vi "record_temp.vi"() -> ()   [LabVIEW 2013]
doc: "Use this template to build a producer/consumer design pattern with events to produce queue items. Use this design pattern instead of the User Interface Event Handler pattern for user interfaces when you want to execute code asynchronously in response to an event without slowing the user interface responsiveness."
uses:
  prog_files_all/ni/labview/examples/Instrument IO/Serial/support/Serial - Settings.ctl
  states_cntrl.ctl
  raw_dat_str.ctl
  temp_ind.ctl
  dts_cntrl.ctl
  rh_ind.ctl
  usr_evnt_main_clstr.ctl
  event_clstr.ctl
  log_dat.ctl
  rh_ind_arry.ctl
  sens_type.ctl
  sens_type_arry_cntrl.ctl
  pibs_clstr.ctl
  sens_type_arry_str_cntrl.ctl
  reg_evnt_ref_clstr.ctl
  labview/power_vi_stm_v13_1_7_22/labview/gen_libs/non_instr/gen_ctls/enums/minor_qsm.ctl
  labview/power_vi_stm_v13_1_7_22/labview/gen_libs/both/gen_ctls/rs232_data_clstr.ctl
  labview/power_vi_stm_v13_1_7_22/labview/gen_libs/non_instr/gen_ctls/enums/state_enum.ctl
  <vilib>/Instr/_visa.llb/VISA Configure Serial Port (Instr).vi
panel:
  out "sens_typ_str _2":T1
  in  "sens_type_8":T2 items=["SHTC3", "SHT3X", "D6T_1A", "HTS221", "AHT20", "ADT7410"]
  in  "sens_type_7":T2 items=["SHTC3", "SHT3X", "D6T_1A", "HTS221", "AHT20", "ADT7410"]
  in  "sens_type_6":T2 items=["SHTC3", "SHT3X", "D6T_1A", "HTS221", "AHT20", "ADT7410"]
  in  "sens_type_5":T2 items=["SHTC3", "SHT3X", "D6T_1A", "HTS221", "AHT20", "ADT7410"]
  in  "sens_type_4":T2 caption="Sensor Type" items=["SHTC3", "SHT3X", "D6T_1A", "HTS221", "AHT20", "ADT7410"]
  in  "sens_type_3":T2 caption="Sensor Type" items=["SHTC3", "SHT3X", "D6T_1A", "HTS221", "AHT20", "ADT7410"]
  in  "sens_type_2":T2 caption="Sensor Type" items=["SHTC3", "SHT3X", "D6T_1A", "HTS221", "AHT20", "ADT7410"]
  in  "sens_type_1":T2 caption="Sensor Type" items=["SHTC3", "SHT3X", "D6T_1A", "HTS221", "AHT20", "ADT7410"]
  out "rh_8":T3 caption="Relative Humidity (%)" format="%#_4g"
  out "sen_8_num":T4 caption="Temp (F)" format="%_4g"
  out "rh_7":T3 caption="Relative Humidity (%)" format="%#_4g"
  out "sen_7_num":T4 caption="Temp (F)" format="%_4g"
  out "rh_6":T3 caption="Relative Humidity (%)" format="%#_4g"
  out "sen_6_num":T4 caption="Temp (F)" format="%_4g"
  out "rh_5":T3 caption="Relative Humidity (%)" format="%#_4g"
  out "sen_5_num":T4 caption="Temp (F)" format="%_4g"
  out "rh_4":T3 caption="Relative Humidity (%)" format="%#_4g"
  out "sen_4_num":T4 caption="Temp (F)" format="%_4g"
  out "sen_3_num":T4 caption="Temp (F)" format="%_4g"
  out "sen_2_num":T4 caption="Temp (F)" format="%_4g"
  out "rh_3":T3 caption="Relative Humidity (%)" format="%#_4g"
  out "rh_2":T3 caption="Relative Humidity (%)" format="%#_4g"
  out "sen_1":T5
  out "sen_1_num":T4 caption="Temp (F)" format="%_4g"
  out "sen_2":T5
  out "sen_3":T5
  out "sen_4":T5
  out "sen_5":T5
  out "sen_6":T5
  out "sen_7":T5
  out "sen_8":T5
  out "rh_1":T3 caption="Relative Humidity (%)" format="%#_4g"
  out "sens_typ_str":T1
  out "sens_type_arry":T6 items=["SHTC3", "SHT3X", "D6T_1A", "HTS221", "AHT20", "ADT7410"]
  in  "regEvntClstr":T7
  in  "user event out":T8
  out "states_ind":T9 caption="State_Ind"
  in  "stop":bool
  in  "tab_cntrl":T10(tab)
  in  "Serial Settings":T11={"baud rate"=19200, "data bits"=8, "parity"=enum."None", "stop bits"=10, "flow control"=0} {"flow control" items=["None"=0, "XON/XOFF"=1, "RTS/CTS"=2, "DTR/DSR"=4]; "stop bits" items=["1.0"=10, "1.5"=15, "2.0"=20]; "data bits" min=5 max=8 step=1; "baud rate" items=["75"=75, "110"=110, "134"=134, "150"=150, "300"=300, "600"=600, "1200"=1200, "1800"=1800, "2400"=2400, "4800"=4800, "7200"=7200, "9600"=9600, "14400"=14400, "19200"=19200, "28800"=28800, "38400"=38400, "56000"=56000, "57600"=57600, "115200"=115200, "128000"=128000, "230400"=230400]}
  in  "VISA resource name":refnum<visa-resource-name>="COM3"
  in  "minor_qsm_qry":bool caption="Use Minor QSM"
  in  "capt_data":bool
  in  "wr_buffr":string="\b"
  in  "dwell_s":u32=60
  in  "auto_capt_data":bool
  in  "delay":u32=10
  out "bytes_at_port":u32
  out "bytes read":u32
  out "Response":string
  in  "small_dwell":u32=3
  in  "chk_bytes_rd":u32=56
  in  "pibs_clstr":T12 {"sens_type_8" items=["SHTC3", "SHT3X", "D6T_1A", "HTS221", "AHT20", "ADT7410"]; "sens_type_7" items=["SHTC3", "SHT3X", "D6T_1A", "HTS221", "AHT20", "ADT7410"]; "sens_type_6" items=["SHTC3", "SHT3X", "D6T_1A", "HTS221", "AHT20", "ADT7410"]; "sens_type_5" items=["SHTC3", "SHT3X", "D6T_1A", "HTS221", "AHT20", "ADT7410"]; "sens_type_4" items=["SHTC3", "SHT3X", "D6T_1A", "HTS221", "AHT20", "ADT7410"]; "sens_type_3" items=["SHTC3", "SHT3X", "D6T_1A", "HTS221", "AHT20", "ADT7410"]; "sens_type_2" items=["SHTC3", "SHT3X", "D6T_1A", "HTS221", "AHT20", "ADT7410"]; "sens_type_1" items=["SHTC3", "SHT3X", "D6T_1A", "HTS221", "AHT20", "ADT7410"]; "rh_8" format="%#_4g"; "sen_8_num" format="%_4g"; "rh_7" format="%#_4g"; "sen_7_num" format="%_4g"; "rh_6" format="%#_4g"; "sen_6_num" format="%_4g"; "rh_5" format="%#_4g"; "sen_5_num" format="%_4g"; "rh_4" format="%#_4g"; "sen_4_num" format="%_4g"; "sen_3_num" format="%_4g"; "sen_2_num" format="%_4g"; "rh_3" format="%#_4g"; "rh_2" format="%#_4g"; "sen_1_num" format="%_4g"; "rh_1" format="%#_4g"}
  in  "create_file":bool
  in  "Save":bool
  in  "Path":path
  out "dts":T13
  out "concatenated string":string
  in  "mult_list":i32(listbox)
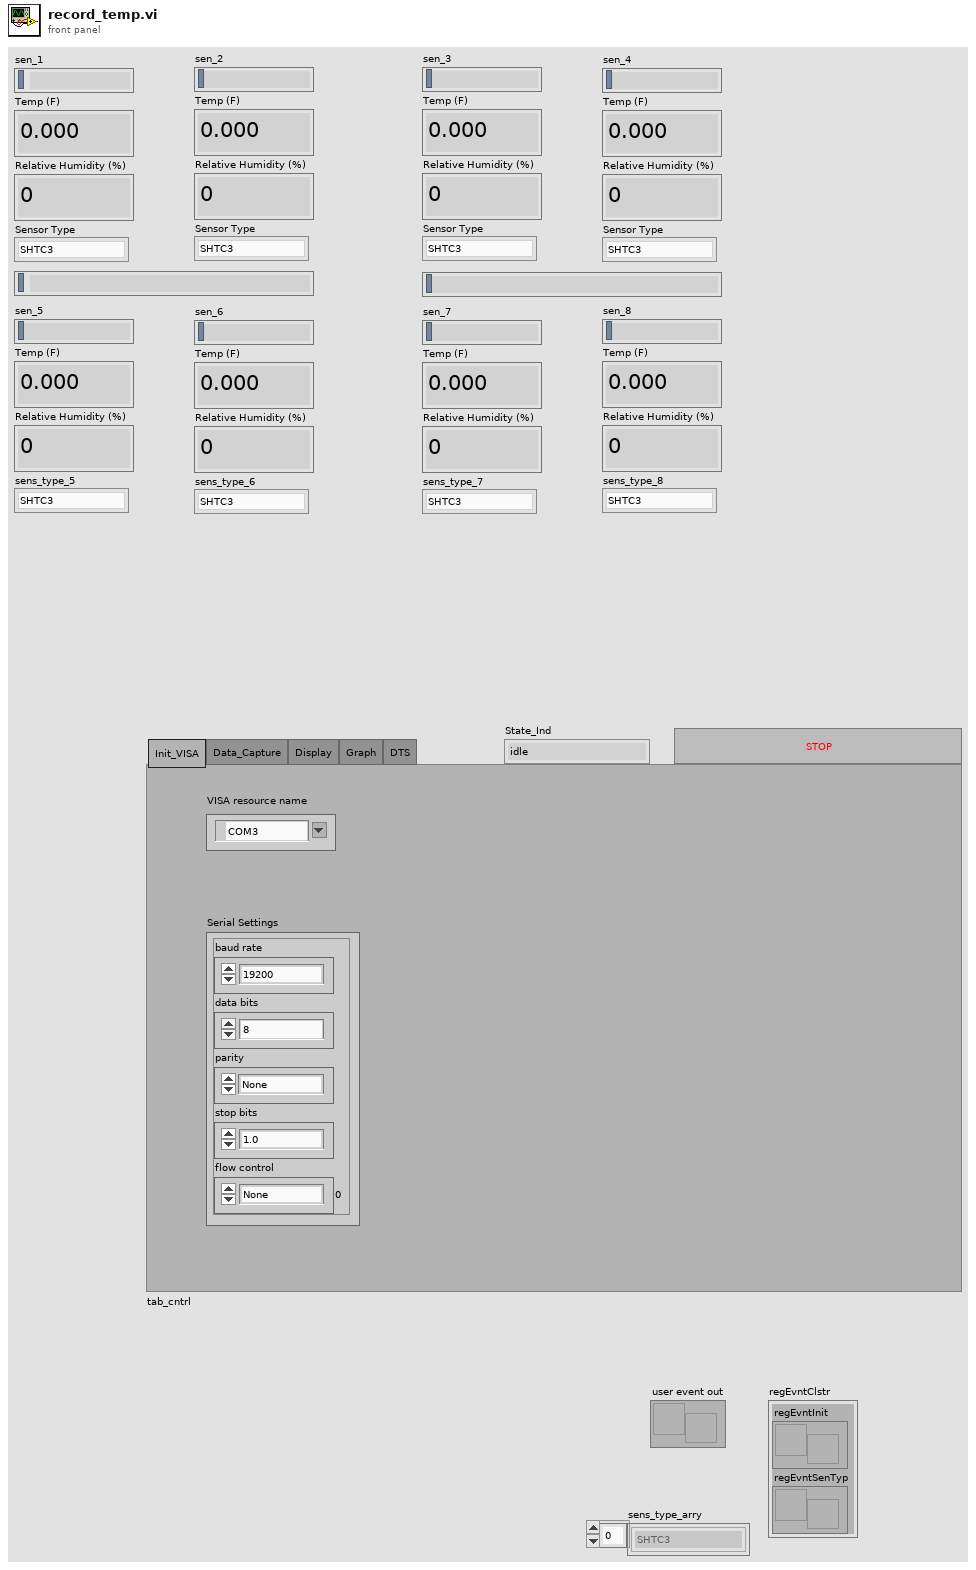
[diagram p1: front panel]
types:
  T1 = typedef "sens_type_arry_str_cntrl.ctl" = string
  T2 = typedef "sens_type.ctl" = u8
  T3 = typedef "rh_ind.ctl" = dbl
  T4 = typedef "temp_ind.ctl" = dbl
  T5 = typedef "raw_dat_str.ctl" = string
  T6 = typedef "sens_type_arry_cntrl.ctl" = T2[]
  T7 = typedef "reg_evnt_ref_clstr.ctl" = cluster{"regEvntInit":refnum<user-event>, "regEvntSenTyp":refnum<user-event>}
  T8 = typedef "usr_evnt_main_clstr.ctl" = refnum<user-event>
  T9 = typedef "states_cntrl.ctl" = enum16{"idle", "exit", "init", "obtain_q", "capt_data", "snd_sens_type", "send_cmd", "capt_wait", "read_data", "chk_bytes_rd", "disp_data", "sav_qry", "sav_dat", "dwell", "small_dwell", "stop_capt_qry", "go_to_minor_qsm", "retr_data", "auto_in_minor_qsm"}
  T10 = enum32{"Init_VISA", "Data_Capture", "Display", "Graph", "DTS"}
  T11 = typedef "Serial - Settings.ctl" = cluster{"baud rate":u32, "data bits":u16, "parity":enum16{"None", "Odd", "Even", "Mark", "Space"}, "stop bits":u16, "flow control":u16}
  T12 = typedef "pibs_clstr.ctl" = cluster{"sens_typ_str":T1, "rh_1":T3, "sen_8":T5, "sen_7":T5, "sen_6":T5, "sen_5":T5, "sen_4":T5, "sen_3":T5, "sen_2":T5, "sen_1_num":T4, "sen_1":T5, "rh_2":T3, "rh_3":T3, "sen_2_num":T4, "sen_3_num":T4, "sen_4_num":T4, "rh_4":T3, "sen_5_num":T4, "rh_5":T3, "sen_6_num":T4, "rh_6":T3, "sen_7_num":T4, "rh_7":T3, "sen_8_num":T4, "rh_8":T3, "sens_type_1":T2, "sens_type_2":T2, "sens_type_3":T2, "sens_type_4":T2, "sens_type_5":T2, "sens_type_6":T2, "sens_type_7":T2, "sens_type_8":T2, "sens_typ_str _2":T1}
  T13 = typedef "dts_cntrl.ctl" = string
  T14 = typedef "minor_qsm.ctl" = cluster{"rs232_comm_q":refnum<queue>, "rs232_data_clstr":T15}
  T15 = typedef "rs232_data_clstr.ctl" = cluster{"state":T16, "connection ID":refnum<k5>, "stop_evnt_loop":bool, "main_q":refnum<queue>, "bytes read":u32, "Response":string, "wr_buffr":string, "bytes_at_port":u32, "visa_rsc_out":refnum<visa-resource-name>, "delay":u32, "sens_type_arry":T6, "chk_bytes_rd":u32}
  T16 = typedef "state_enum.ctl" = enum16{"idle", "exit", "obtain_q", "init", "create_file", "pik_sampl_mode", "init_instr_finite", "init_instr_cont", "update_file_path", "change_v_setting", "change _i_range", "turn_on_cur_qry", "turn_on_tst_cur", "dwell", "temp_stb_dwell", "meas", "v_set_qry", "range_qry", "save_data", "display_data", "cmd_proxy_state", "setting_proxy_state", "turn_off_tst_cur", "turn_off_curr_to_stop", "max_turn_off_trials_qry", "exit_prog", "max_trials_qry", "empty_str_qry", "man_cmd_qry", "man_cmd_qry_after_x_times", "cyc_qry", "turn_on_tcm", "turn_off_tcm", "chk_for_tcm", "max_trials_for_tcm", "turn_on_init_tcm", "srch_for_all_files", "strt_pdf_file", "append_pic", "append_header", "append_new_page", "pics_done_qry", "close_pdf_file", "set_cal_volt", "meas_cal_volt", "incr_voltage", "incr_cur_g1", "incr_cur_g2", "first_last_cyc_qry", "compare_results", "update_params", "cont_meas", "set_first_cur", "test_done_qry", "init_m3_temp_qry", "m3_diff_temp_qry", "temp_rched_qry", "set_init_oven_temp", "oven_temp_dwell", "update_oven_settings", "meas_oven_temp", "oven_temp_diff", "get_dat_from_vis", "ret_dat_from_cdaq", "ret_dat_from_ps", "close_cont_daqs", "cyc_trig_qry", "hot_temp_trig_qry", "cold_temp_trig_qry", "amb_temp_trig_qry", "both_temps_trig_qry", "temp_cond_hot_qry", "temp_cond_cold_qry", "temp_cond_amb_qry", "dur_strt_qry", "dur_end_qry", "daq_per_trig_qry", "src_type_qry", "turn_on_ps_1", "turn_off_ps_1", "turn_on_ps_2", "turn_off_ps_2", "data_type_qry", "user_stop_qry", "ret_data", "stm_snd_to_client", "strt_stm_listen", "snd_cmd", "capt_wait", "read_data", "chk_bytes_rd"}
  T17 = typedef "event_clstr.ctl" = cluster{"states":T9, "bytes read":u32, "Response":string, "wr_buffr":string, "bytes_at_port":u32, "temp_clstr":T18, "logTable in":string[][][], "mult_list":i32, "log_tabl_row_cnt":u64, "above_row_7":bool, "sens_type":T2, "sens_type_arry":T6, "pibs_clstr":T12, "dts":T13}
  T18 = typedef "log_dat.ctl" = cluster{"sen_4_num":T4, "sen_3_num":T4, "sen_2_num":T4, "sen_1_num":T4, "sen_8_num":T4, "sen_7_num":T4, "sen_6_num":T4, "sen_5_num":T4, "dts":string, "sen_4":string, "sen_3":string, "sen_2":string, "sen_1":string, "sen_8":string, "sen_7":string, "sen_6":string, "sen_5":string, "temp_f_arry":T4[], "sens_dat_raw_arry":string[], "raw_dat":string, "rh_arry":T19, "rh_1":T3, "rh_0":T3, "rh_3":T3, "rh_2":T3, "rh_5":T3, "rh_4":T3, "rh_7":T3, "rh_6":T3}
  T19 = typedef "rh_ind_arry.ctl" = T3[]
  T20 = enum16{"open", "replace", "create", "open or create", "replace or create", "replace or create with confirmation"}
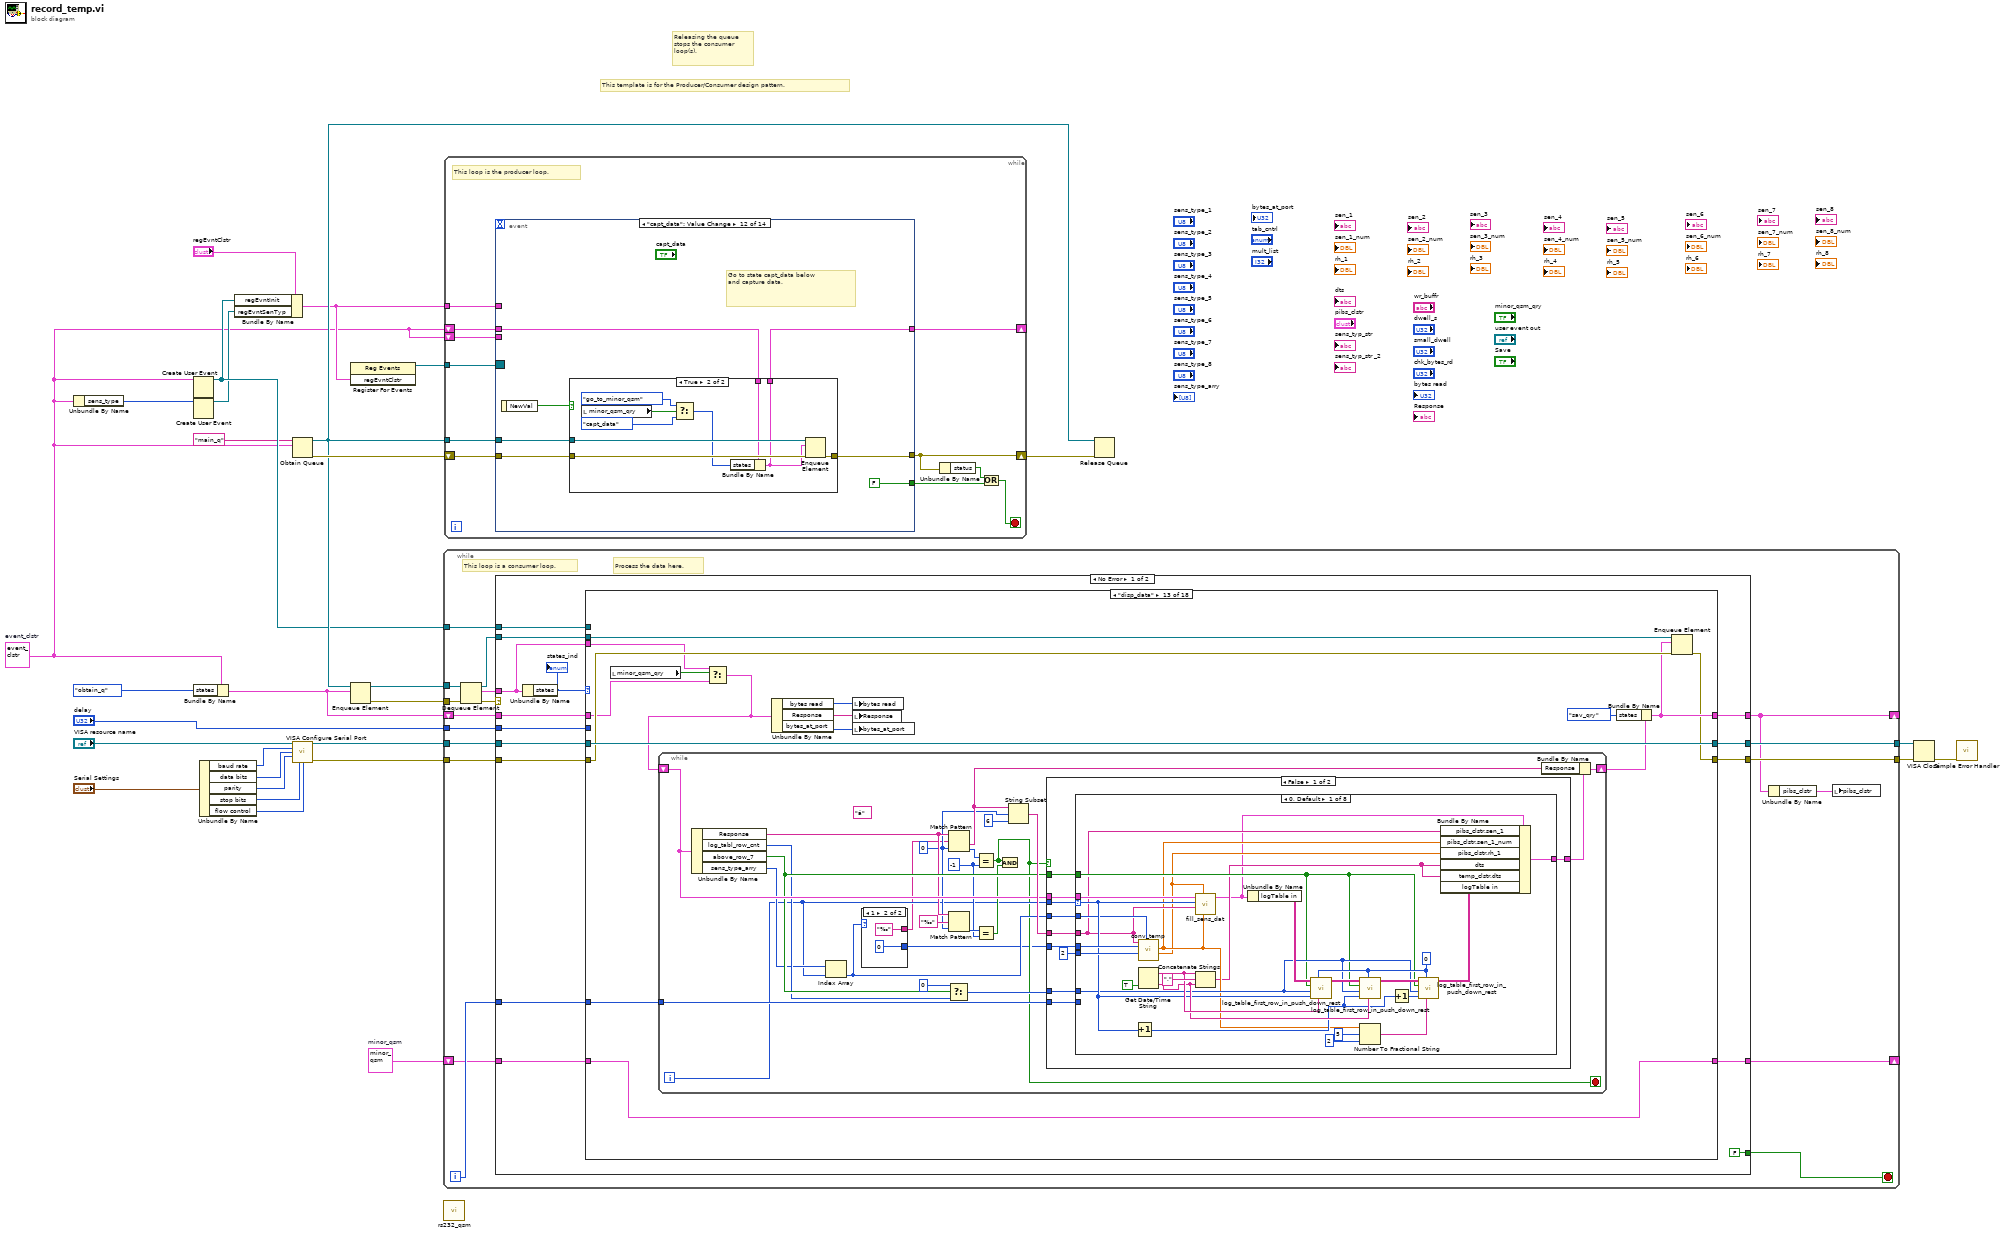
[diagram p0: block diagram]
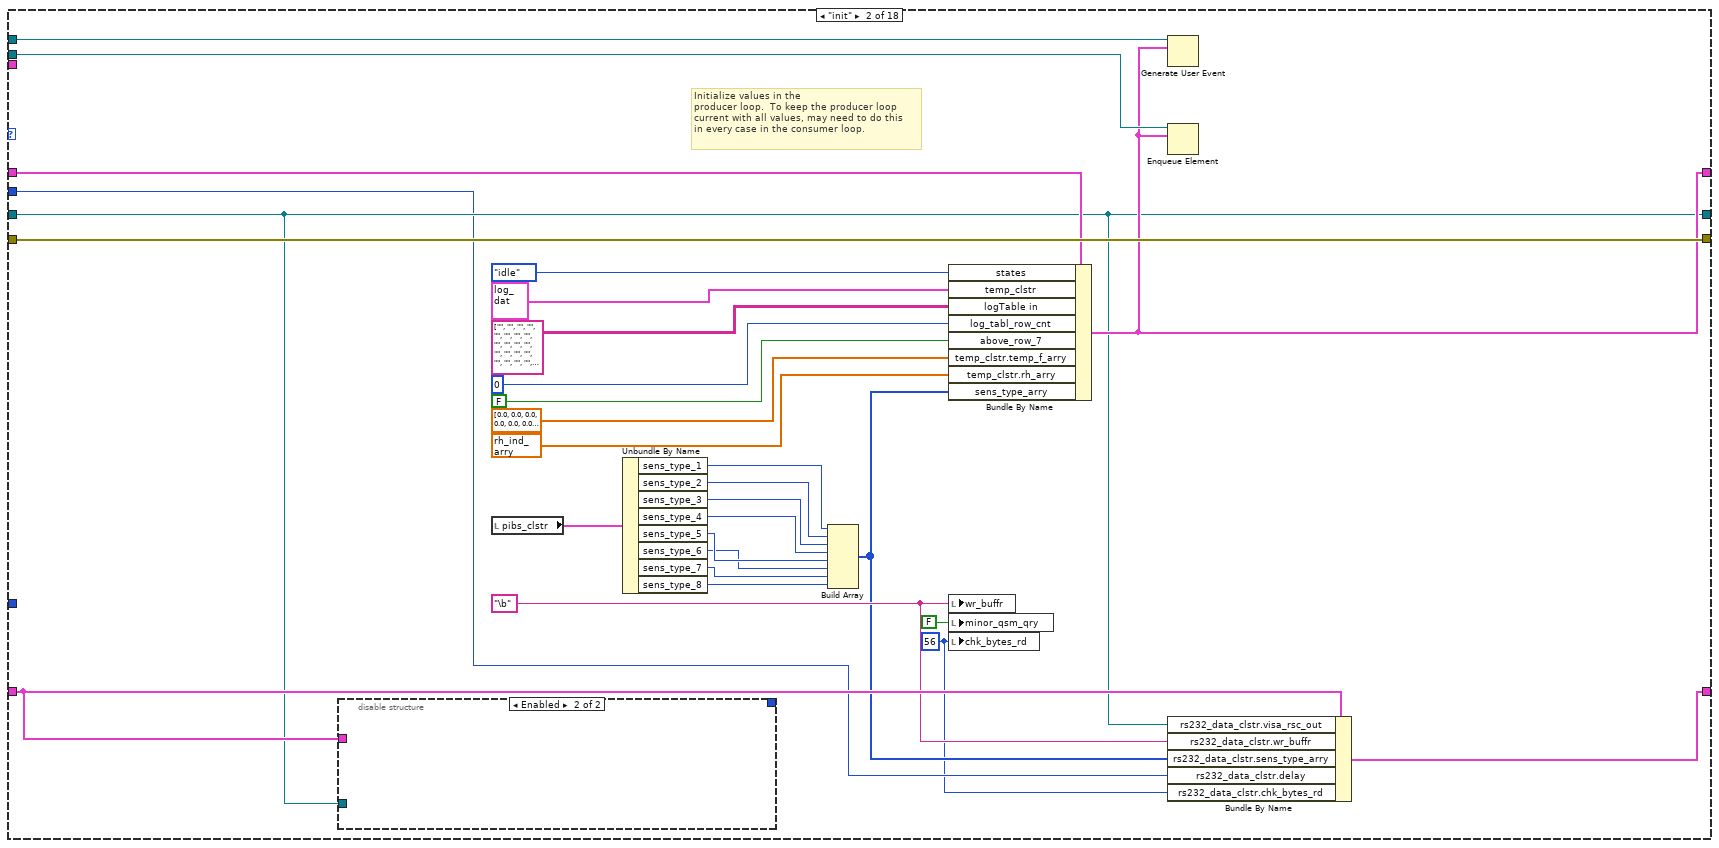
[diagram p3: hidden frame]
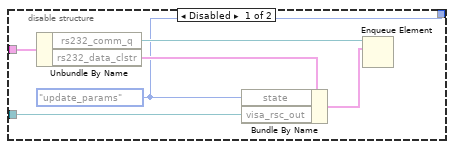
[diagram p4: hidden frame]
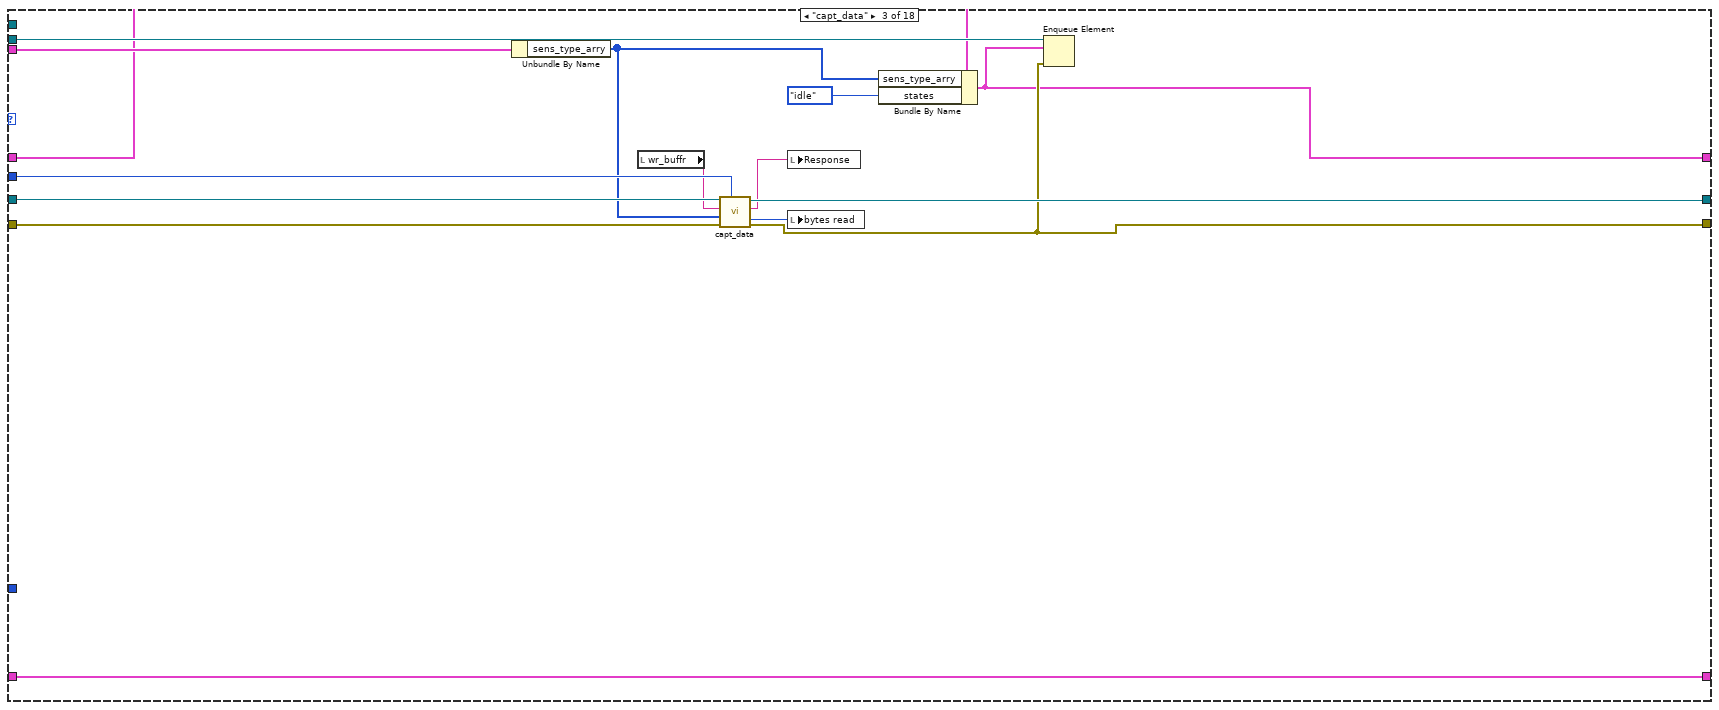
[diagram p5: hidden frame]
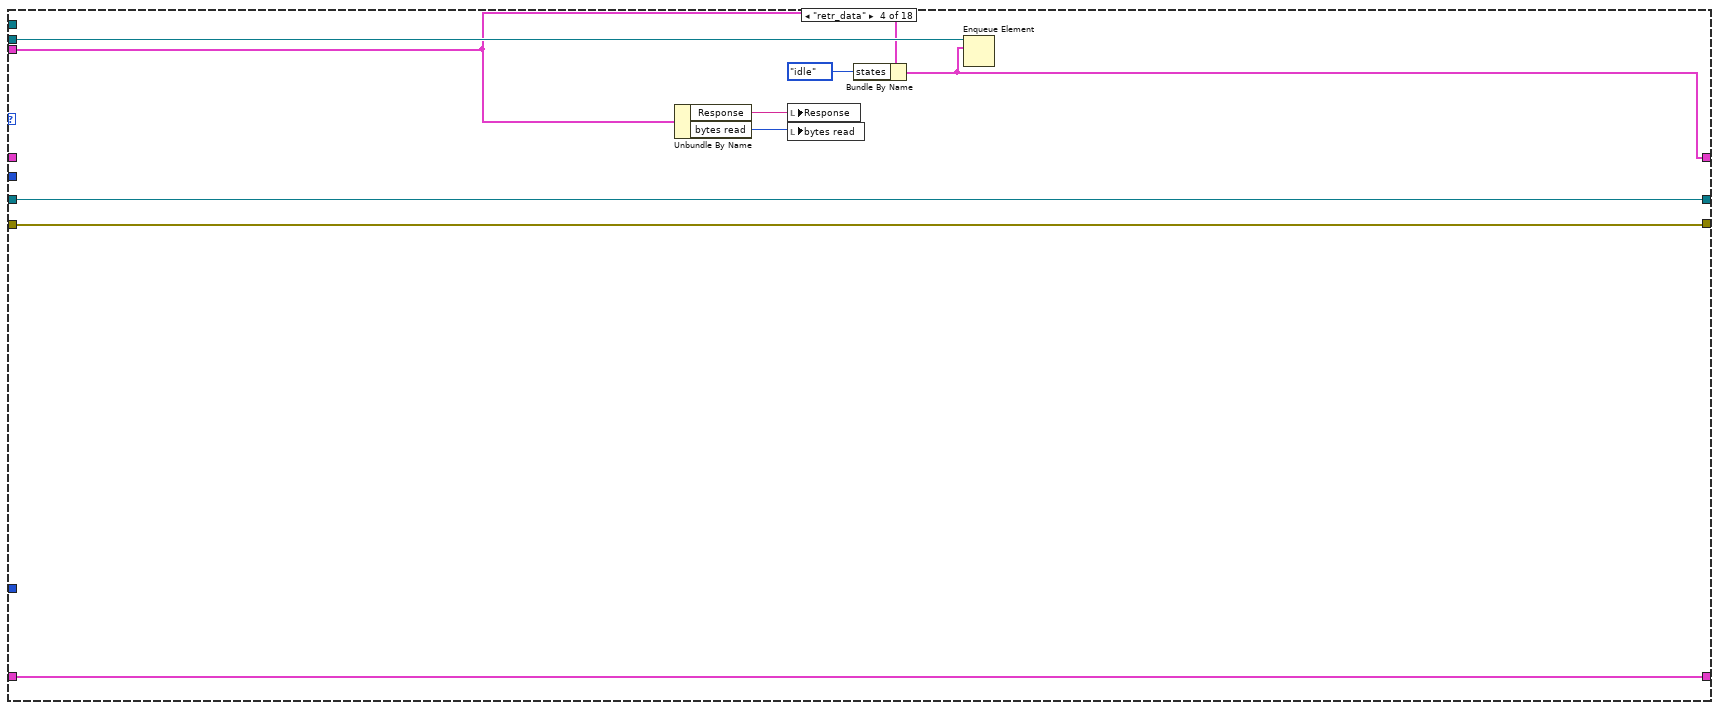
[diagram p6: hidden frame]
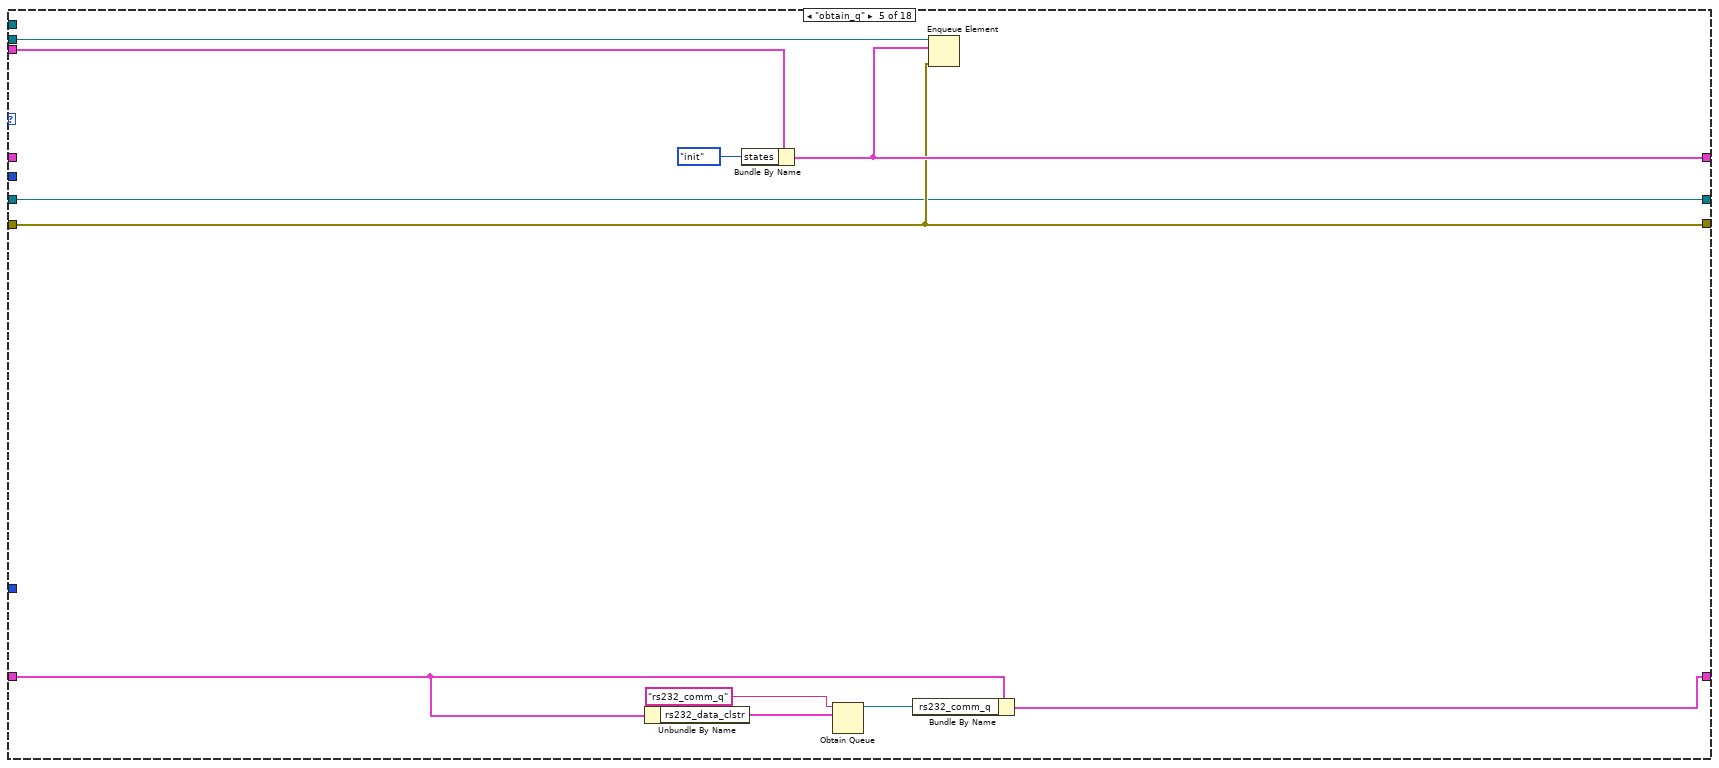
[diagram p7: hidden frame]
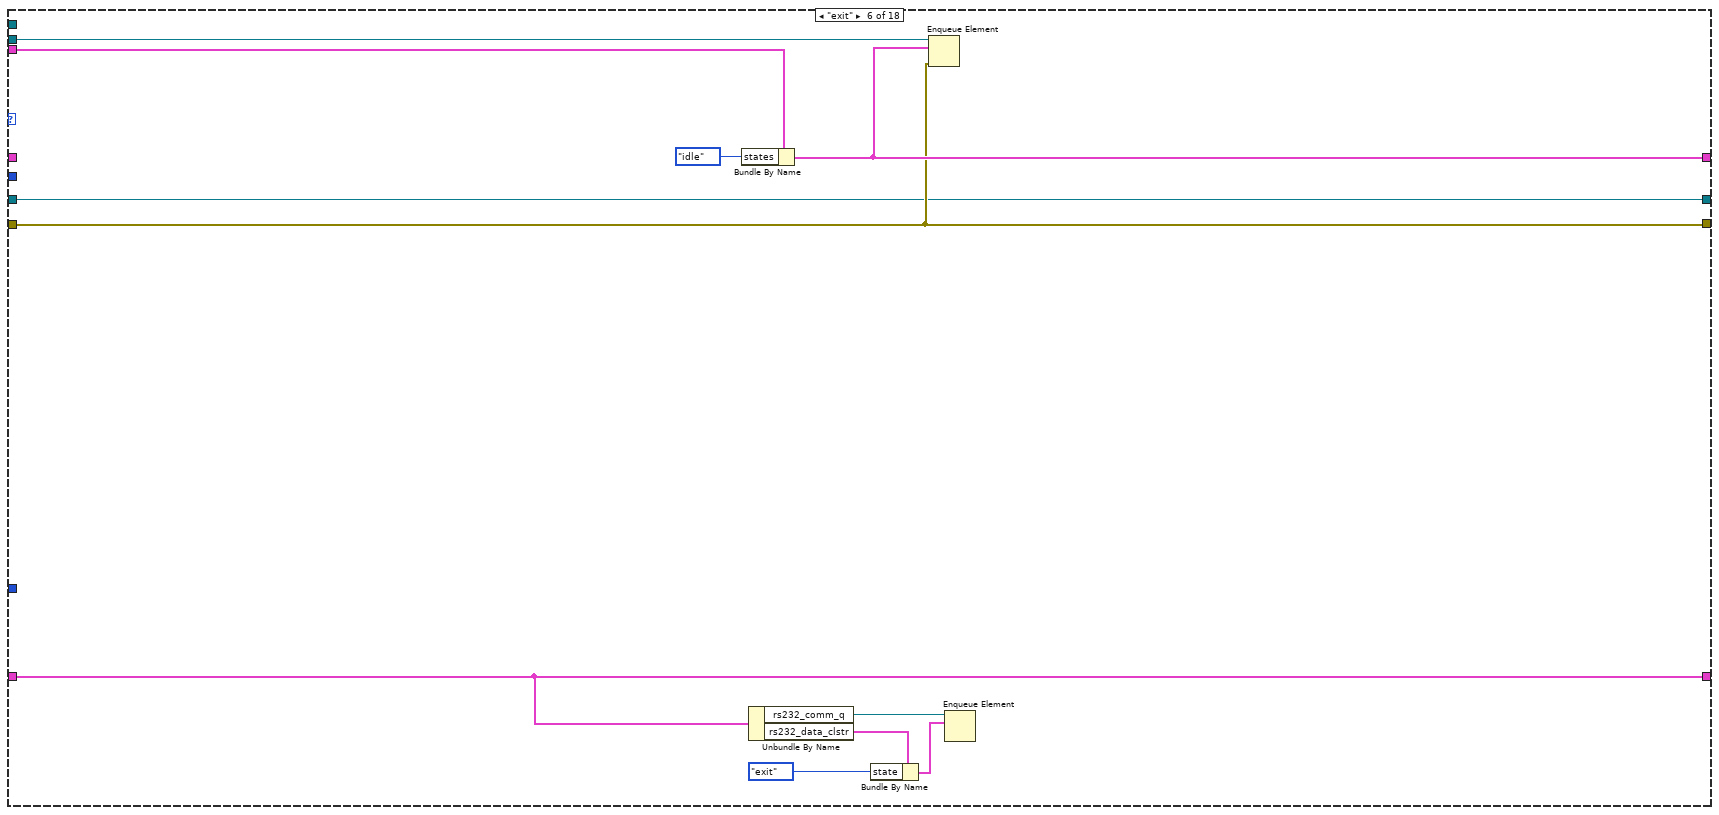
[diagram p8: hidden frame]
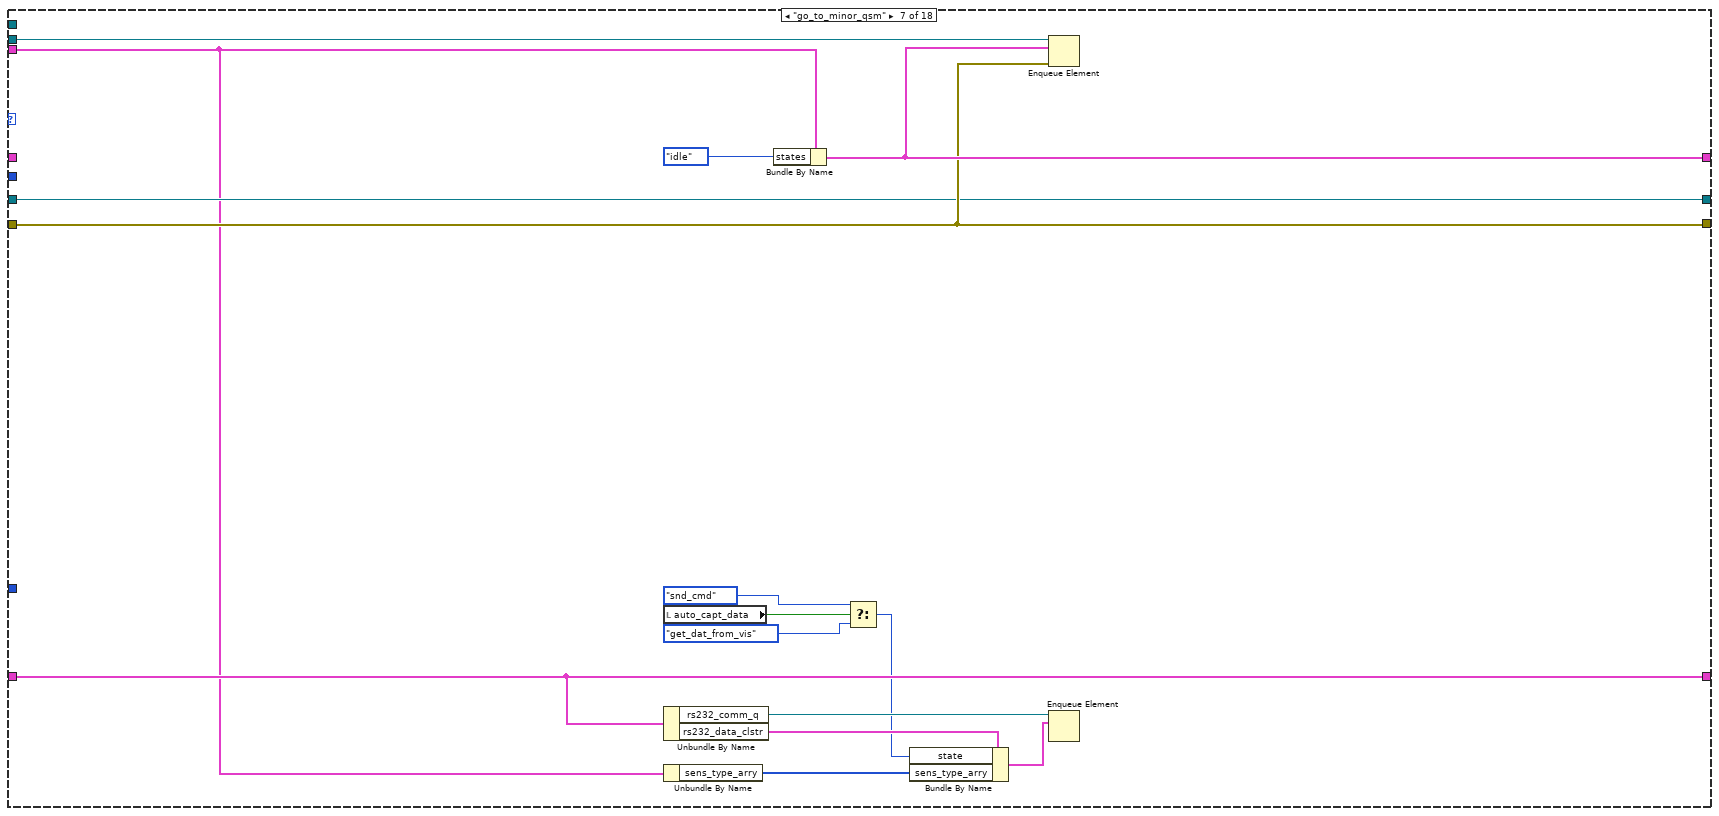
[diagram p9: hidden frame]
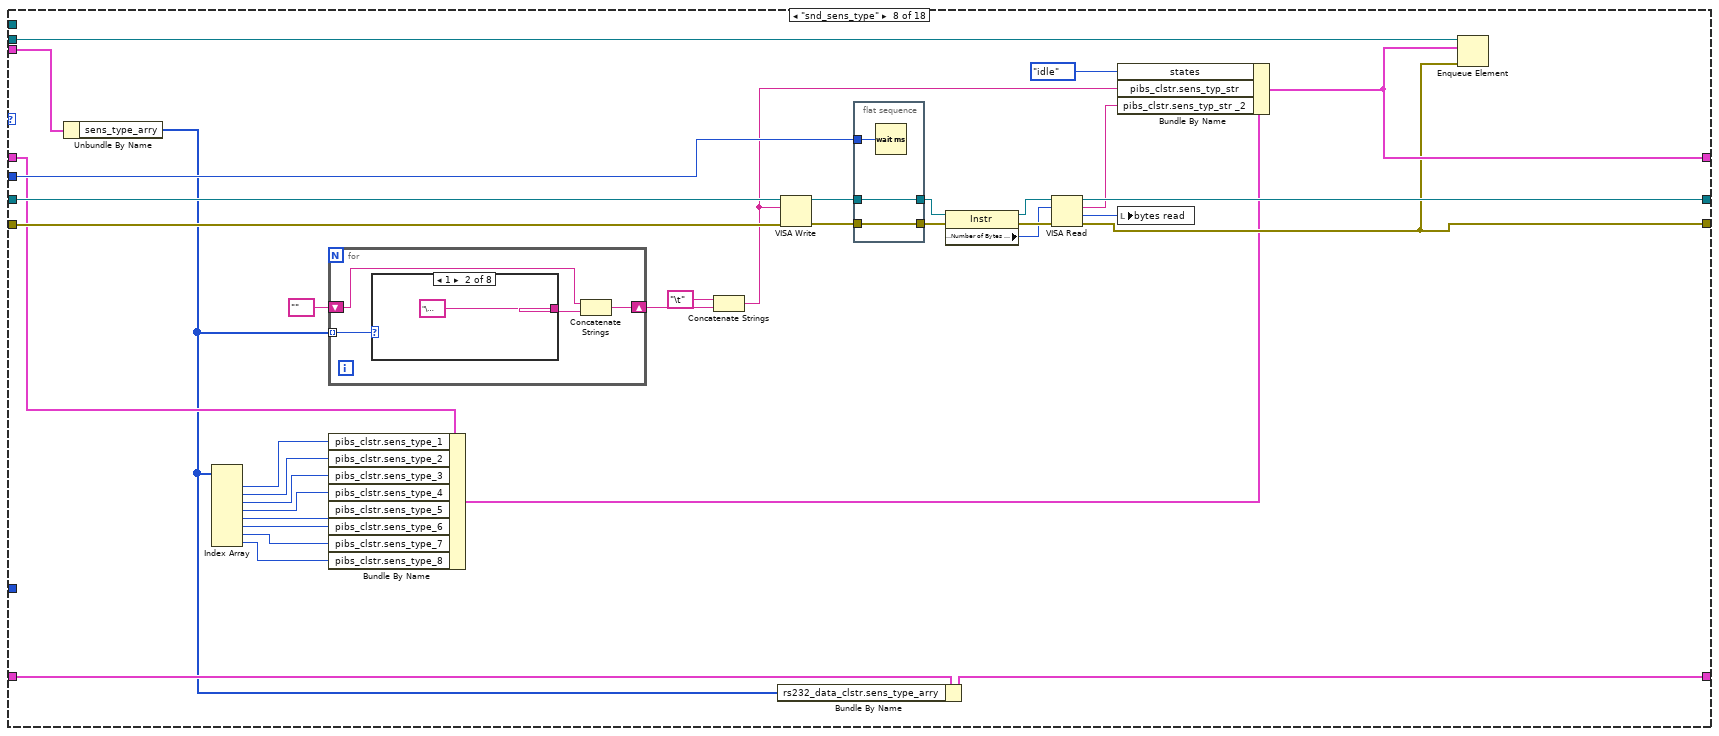
[diagram p10: hidden frame]
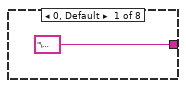
[diagram p11: hidden frame]
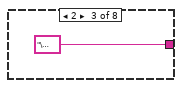
[diagram p12: hidden frame]
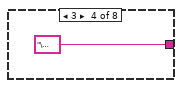
[diagram p13: hidden frame]
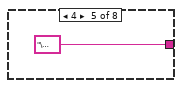
[diagram p14: hidden frame]
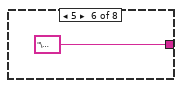
[diagram p15: hidden frame]
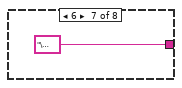
[diagram p16: hidden frame]
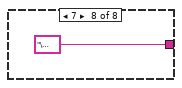
[diagram p17: hidden frame]
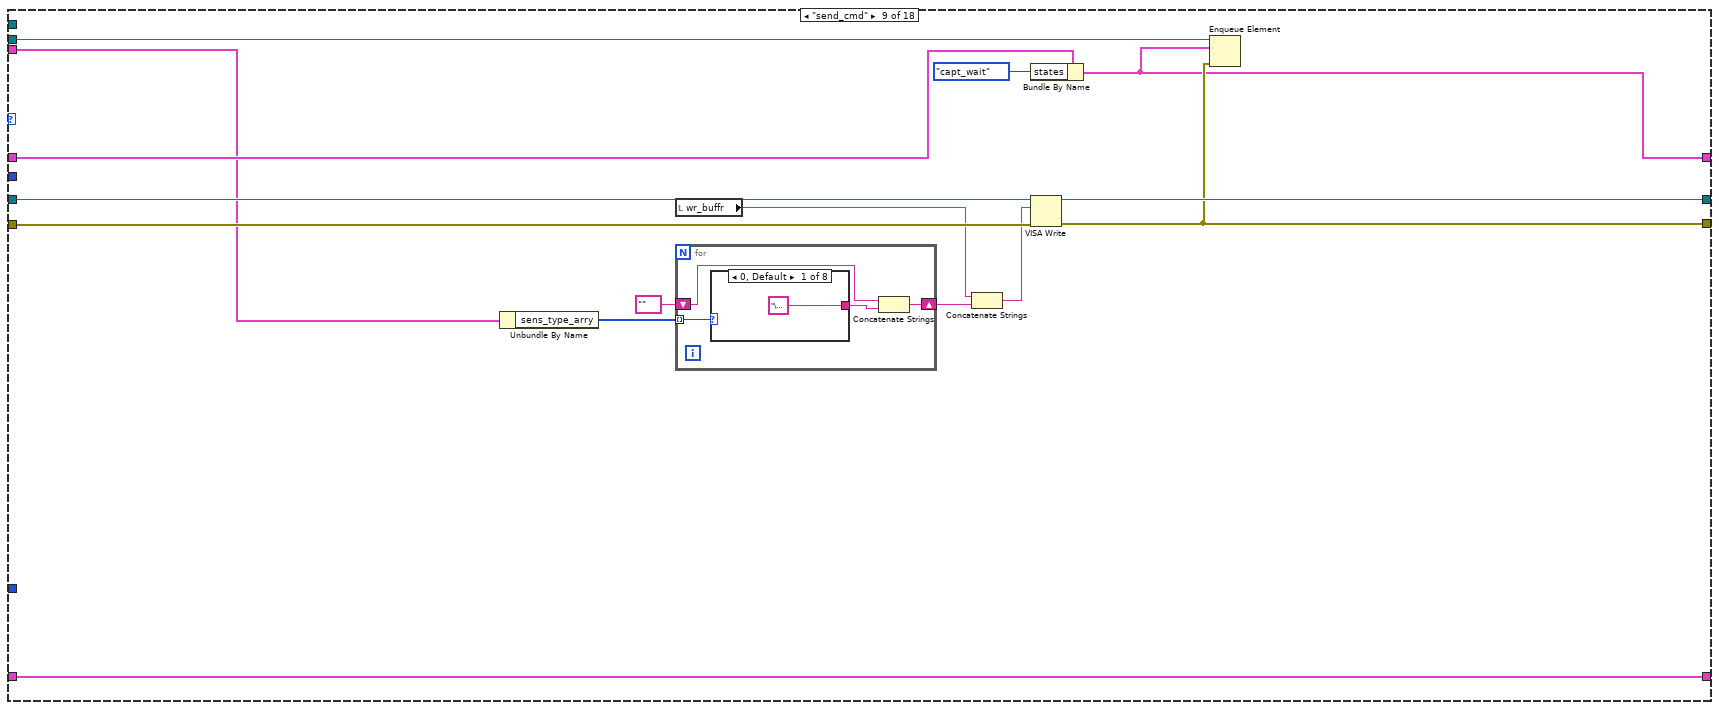
[diagram p18: hidden frame]
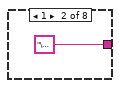
[diagram p19: hidden frame]
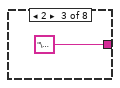
[diagram p20: hidden frame]
diagram:
  w3 = T14 {"rs232_comm_q"=refnum, "rs232_data_clstr"={"state"=enum."idle", "connection ID"=refnum, "stop_evnt_loop"=FALSE, "main_q"=refnum, "bytes read"=0, "Response"="", "wr_buffr"="", "bytes_at_port"=0, "visa_rsc_out"="", "delay"=0, "sens_type_arry"=[], "chk_bytes_rd"=0}}  # minor_qsm
  w5 = T17 {"states"=enum."init", "bytes read"=7, "Response"="á7Mìhc\u000b", "wr_buffr"="\b", "bytes_at_port"=0, "temp_clstr"={"sen_4_num"=0.0, "sen_3_num"=0.0, "sen_2_num"=0.0, "sen_1_num"=0.0, "sen_8_num"=0.0, "sen_7_num"=0.0, "sen_6_num"=0.0, "sen_5_num"=0.0, "dts"="", "sen_4"="", "sen_3"="", "sen_2"="", "sen_1"="", "sen_8"="", "sen_7"="", "sen_6"="", "sen_5"="", "temp_f_arry"=[], "sens_dat_raw_arry"=[], "raw_dat"="", "rh_arry"=[], "rh_1"=0.0, "rh_0"=0.0, "rh_3"=0.0, "rh_2"=0.0, "rh_5"=0.0, "rh_4"=0.0, "rh_7"=0.0, "rh_6"=0.0}, "logTable in"=[], "mult_list"=0, "log_tabl_row_cnt"=0, "above_row_7"=FALSE, "sens_type"=0, "sens_type_arry"=[], "pibs_clstr"={"sens_typ_str"="", "rh_1"=0.0, "sen_8"="", "sen_7"="", "sen_6"="", "sen_5"="", "sen_4"="", "sen_3"="", "sen_2"="", "sen_1_num"=0.0, "sen_1"="", "rh_2"=0.0, "rh_3"=0.0, "sen_2_num"=0.0, "sen_3_num"=0.0, "sen_4_num"=0.0, "rh_4"=0.0, "sen_5_num"=0.0, "rh_5"=0.0, "sen_6_num"=0.0, "rh_6"=0.0, "sen_7_num"=0.0, "rh_7"=0.0, "sen_8_num"=0.0, "rh_8"=0.0, "sens_type_1"=0, "sens_type_2"=0, "sens_type_3"=0, "sens_type_4"=0, "sens_type_5"=0, "sens_type_6"=0, "sens_type_7"=0, "sens_type_8"=0, "sens_typ_str _2"=""}, "dts"=""}  # event_clstr
  # "Releasing the queue stops the consumer loop(s)."
  # "This template is for the Producer/Consumer design pattern."
  n1 = Unbundle By Name(w5) -> ("sens_type"=w7:T2)
  n2 = Create User Event(user event datatype=w5) -> (user event=w10:refnum<user-event>)  [unwired: 1 in, 1 out]
  n3 = Create User Event(user event datatype=w7) -> (user event=w9:refnum<user-event>)  [unwired: 1 in, 1 out]
  n4 = Bundle By Name(cluster=w5, "states"=states_cntrl."obtain_q") -> (w2:T17)
  n5 = Unbundle By Name("Serial Settings") -> ("baud rate"=w11:u32, "data bits"=w24:u16, "parity"=w25:enum16{"None", "Odd", "Even", "Mark", "Space"}, "stop bits"=w26:u16, "flow control"=w27:u16)
  n6 = Bundle By Name(cluster="regEvntClstr", "regEvntInit"=w10, "regEvntSenTyp"=w9) -> (w6:T7)
  n7 = Obtain Queue(name (unnamed)="main_q", element data type=w5) -> (queue out=w16:refnum<queue>, error out=w29:errorcluster)  [unwired: 3 in, 1 out]
  n8 = call-poly "VISA Configure Serial Port"("VISA resource name"="VISA resource name", "baud rate (9600)"=w11, "data bits (8)"=w24, "parity (0:none)"=w25, "stop bits (10: 1 bit)"=w26, "flow control (0:none)"=w27) -> ("VISA resource name out"=w21:refnum<visa-resource-name>, "error out"=w17:errorcluster)  [unwired: 3 in, 5 out]
  n9 = register-events(w6) -> (reference out=w12:refnum<event-registration>)  [unwired: 2 in, 1 out]
  n10 = Enqueue Element(queue=w16, element=w2) -> (queue out=w15:refnum<queue>, error out=w14:errorcluster)  [unwired: 2 in, 1 out]
  n11 = while {
    tunnel: w15 -> [w47]
    tunnel: w21 -> [w44]
    tunnel: [w43] -> w19
    tunnel: [w42] -> w18
    tunnel: w17 -> [w41]
    tunnel: w14 -> [w39]
    tunnel: "delay" -> [w38]
    shift-right: [w34] -> _
    shift-left: w2 -> [w37]
    tunnel: w10 -> [w35]
    shift-right: [w30] -> _
    shift-left: w3 -> [w31]
    i -> [w36]
    stop <- w32 stop-if-true
    # "Process the data here."
    # "This loop is a consumer loop."
    n12 = Dequeue Element(queue=w47, error in (no error)=w39) -> (queue out=w40:refnum<queue>, element=w45:T17, error out=w46:errorcluster)  [unwired: 1 in, 1 out]
    n13 = case shown="No Error" w46 {
      tunnel: w45 -> [w55 _]
      tunnel: [FALSE TRUE] -> w32
      tunnel: w44 -> [w60 w599]
      tunnel: [w59 w599] -> w43
      tunnel: [w58 w598] -> w42
      tunnel: w41 -> [w57 w598]
      tunnel: w40 -> [w56 _]
      tunnel: w38 -> [w54 _]
      tunnel: w37 -> [w53 w597]
      tunnel: [w52 w597] -> w34
      tunnel: w36 -> [w51 _]
      tunnel: w35 -> [w50 _]
      tunnel: w31 -> [w49 w596]
      tunnel: [w48 w596] -> w30
      frame No Error {
        n14 = Unbundle By Name(w55) -> ("states"=w62:T9)
        "states_ind" <- w62
        n15 = case shown="\"disp_data\"" w62 {
          tunnel: w60 -> [w65 w72 w116 w118 w129 w141 w157 w195 w227 w249 w262 w277 w293 w507 w521 w564 w579 w594]
          tunnel: [w65 w72 w115 w118 w129 w141 w157 w182 w225 w247 w260 w277 w293 w507 w521 w562 w577 w594] -> w59
          tunnel: [w66 w95 w112 w117 w130 w142 w158 w181 w222 w244 w259 w276 w286 w508 w522 w559 w574 w593] -> w58
          tunnel: w57 -> [w66 w95 w113 w117 w130 w142 w158 w193 w226 w248 w261 w276 w292 w509 w523 w563 w578 w593]
          tunnel: w56 -> [_ w85 w114 w125 w136 w147 w162 w194 w223 w245 w265 w278 w294 w511 w525 w560 w575 w595]
          tunnel: w55 -> [_ _ w108 w122 w133 w144 w153 w176 w215 _ _ _ w281 _ _ _ _ _]
          tunnel: w54 -> [_ w69 w110 _ _ _ _ w191 _ w243 _ _ _ _ _ _ _ _]
          tunnel: w53 -> [w64 w94 w103 _ _ _ _ w175 w220 w241 w254 w269 w280 w513 w519 w555 w570 w588]
          tunnel: [w64 w84 w109 w123 w134 w145 w160 w190 w221 w242 w255 w270 w288 w510 w524 w556 w571 w589] -> w52
          tunnel: w51 -> [_ _ _ _ _ _ _ _ _ _ _ _ w285 _ _ _ _ _]
          tunnel: w50 -> [_ w86 _ _ _ _ _ _ _ _ _ _ _ _ _ _ _ _]
          tunnel: w49 -> [w63 w74 w107 w121 w132 w143 w159 w165 w213 w240 w253 w268 w283 w506 w518 w554 w569 w587]
          tunnel: [w63 w73 w107 w121 w127 w143 w159 w164 w213 w240 w253 w268 w283 w506 w518 w554 w569 w587] -> w48
          frame "idle", Default {
          }
          frame "init" {
            w67 = u32 56 ("chk_bytes_rd")
            w71 = "\b" ("wr_buffr")
            # "Initialize values in the\nproducer loop.  To keep the producer loop\ncurrent with all values, may need to do this\nin every case in the consumer loop."
            n16 = disable-structure shown="Enabled" {
              disable-tunnel: w74 -> [w98 _]
              disable-tunnel: [w97 _] -> _
              disable-tunnel: w72 -> [w96 _]
              frame Disabled {
                w97 = state_enum."update_params" ("state")
                n17 = Unbundle By Name(w98) -> ("rs232_comm_q"=w101:refnum<queue>, "rs232_data_clstr"=w100:T15)
                n18 = Bundle By Name(cluster=w100, "state"=w97, "visa_rsc_out"=w96) -> (w99:T15)
                n19 = Enqueue Element(queue=w101, element=w99) -> ()  [unwired: 2 in, 3 out]
              }
              frame Enabled {
              }
            }
            n20 = local read "pibs_clstr"() -> (w83:T12)
            n21 = Unbundle By Name(w83) -> ("sens_type_1"=w82:T2, "sens_type_2"=w81:T2, "sens_type_3"=w80:T2, "sens_type_4"=w79:T2, "sens_type_5"=w78:T2, "sens_type_6"=w77:T2, "sens_type_7"=w76:T2, "sens_type_8"=w75:T2)
            n22 = Build Array(w82, w81, w80, w79, w78, w77, w76, w75) -> (w70:T2[])
            n23 = Bundle By Name(cluster=w94, "states"=states_cntrl."idle", "temp_clstr"=T18 {"sen_4_num"=6.0, "sen_3_num"=0.0, "sen_2_num"=0.0, "sen_1_num"=0.0, "sen_8_num"=0.0, "sen_7_num"=0.0, "sen_6_num"=0.0, "sen_5_num"=0.0, "dts"="", "sen_4"="", "sen_3"="", "sen_2"="", "sen_1"="", "sen_8"="", "sen_7"="", "sen_6"="", "sen_5"="", "temp_f_arry"=[0.0, 0.0, 0.0, 0.0, 0.0, 0.0, 0.0, 0.0], "sens_dat_raw_arry"=["", "", "", "", "", "", "", " "], "raw_dat"="", "rh_arry"=[], "rh_1"=0.0, "rh_0"=0.0, "rh_3"=0.0, "rh_2"=0.0, "rh_5"=0.0, "rh_4"=0.0, "rh_7"=0.0, "rh_6"=0.0}, "logTable in"=string[][][] [[["", "", "", "", "", "", "", "", "", ""], ["", "", "", "", "", "", "", "", "", ""], ["", "", "", "", "", "", "", "", "", ""], ["", "", "", "", "", "", "", "", "", ""], ["", "", "", "", "", "", "", "", "", ""], ["", "", "", "", "", "", "", "", "", ""], ["", "", "", "", "", "", "", "", "", " "]]], "log_tabl_row_cnt"=u64 0, "above_row_7"=FALSE, "temp_clstr.temp_f_arry"=T4[] [0.0, 0.0, 0.0, 0.0, 0.0, 0.0, 0.0, 0.0], "temp_clstr.rh_arry"=T19 [0.0, 0.0, 0.0, 0.0, 0.0, 0.0, 0.0, 0.0], "sens_type_arry"=w70) -> (w84:T17)
            n24 = local write "wr_buffr"(w71) -> ()
            n25 = local write "minor_qsm_qry"(FALSE ("minor_qsm_qry")) -> ()
            n26 = local write "chk_bytes_rd"(w67) -> ()
            n27 = Generate User Event(user event=w86, event data cluster=w84) -> ()  [unwired: 2 in, 2 out]
            n28 = Enqueue Element(queue=w85, element=w84) -> ()  [unwired: 2 in, 3 out]
            n29 = Bundle By Name(cluster=w74, "rs232_data_clstr.visa_rsc_out"=w72, "rs232_data_clstr.wr_buffr"=w71, "rs232_data_clstr.sens_type_arry"=w70, "rs232_data_clstr.delay"=w69, "rs232_data_clstr.chk_bytes_rd"=w67) -> (w73:T14)
          }
          frame "capt_data" {
            n30 = Unbundle By Name(w108) -> ("sens_type_arry"=w102:T6)
            n31 = local read "wr_buffr"() -> (w104:string)
            n32 = call "capt_data.vi"("delay before read (ms)"=w110, "error in (no error)"=w113, "sens_type_arry"=w102, "wr_buffr"=w104, "VISA Refnum in"=w116) -> ("error out"=w112:errorcluster, "bytes read"=w105:u32, "Response"=w106:string, "VISA Refnum out"=w115:refnum<visa-resource-name>)  [unwired: 3 in]
            n33 = local write "Response"(w106) -> ()
            n34 = local write "bytes read"(w105) -> ()
            n35 = Bundle By Name(cluster=w103, "sens_type_arry"=w102, "states"=states_cntrl."idle") -> (w109:T17)
            n36 = Enqueue Element(queue=w114, element=w109, error in (no error)=w112) -> ()  [unwired: 1 in, 3 out]
          }
          frame "retr_data" {
            n37 = Unbundle By Name(w122) -> ("Response"=w120:string, "bytes read"=w119:u32)
            n38 = local write "Response"(w120) -> ()
            n39 = local write "bytes read"(w119) -> ()
            n40 = Bundle By Name(cluster=w122, "states"=states_cntrl."idle") -> (w123:T17)
            n41 = Enqueue Element(queue=w125, element=w123) -> ()  [unwired: 2 in, 3 out]
          }
          frame "obtain_q" {
            n42 = Unbundle By Name(w132) -> ("rs232_data_clstr"=w128:T15)
            n43 = Bundle By Name(cluster=w133, "states"=states_cntrl."init") -> (w134:T17)
            n44 = Obtain Queue(name (unnamed)="rs232_comm_q", element data type=w128) -> (queue out=w126:refnum<queue>)  [unwired: 3 in, 2 out]
            n45 = Bundle By Name(cluster=w132, "rs232_comm_q"=w126) -> (w127:T14)
            n46 = Enqueue Element(queue=w136, element=w134, error in (no error)=w130) -> ()  [unwired: 1 in, 3 out]
          }
          frame "exit" {
            n47 = Bundle By Name(cluster=w144, "states"=states_cntrl."idle") -> (w145:T17)
            n48 = Unbundle By Name(w143) -> ("rs232_comm_q"=w140:refnum<queue>, "rs232_data_clstr"=w139:T15)
            n49 = Bundle By Name(cluster=w139, "state"=state_enum."exit") -> (w137:T15)
            n50 = Enqueue Element(queue=w147, element=w145, error in (no error)=w142) -> ()  [unwired: 1 in, 3 out]
            n51 = Enqueue Element(queue=w140, element=w137) -> ()  [unwired: 2 in, 3 out]
          }
          frame "go_to_minor_qsm" {
            n52 = local read "auto_capt_data"() -> (w151:bool)
            n53 = Unbundle By Name(w159) -> ("rs232_comm_q"=w156:refnum<queue>, "rs232_data_clstr"=w155:T15)
            n54 = Unbundle By Name(w153) -> ("sens_type_arry"=w152:T6)
            n55 = Bundle By Name(cluster=w153, "states"=states_cntrl."idle") -> (w160:T17)
            n56 = Select(t=state_enum."snd_cmd", s=w151, f=state_enum."get_dat_from_vis" ("state")) -> (s? t:f=w148:T16)
            n57 = Bundle By Name(cluster=w155, "state"=w148, "sens_type_arry"=w152) -> (w154:T15)
            n58 = Enqueue Element(queue=w162, element=w160, error in (no error)=w158) -> ()  [unwired: 1 in, 3 out]
            n59 = Enqueue Element(queue=w156, element=w154) -> ()  [unwired: 2 in, 3 out]
          }
          frame "snd_sens_type" {
            n60 = Unbundle By Name(w176) -> ("sens_type_arry"=w163:T6)
            n61 = Index Array(array=w163) -> (element #1=w174:T2, element #2=w173:T2, element #3=w172:T2, element #4=w171:T2, element #5=w170:T2, element #6=w169:T2, element #7=w168:T2, element #8=w167:T2)  [unwired: 8 in]
            n62 = for {
              shift-right: [w200] -> w187
              shift-left: "" -> [w201]
              tunnel: w163 -> [w198] mode=indexing
              n63 = case shown="1" w198 {
                tunnel: ["\u0000" "\u0001" "\u0002" "\u0003" "\u0004" "\u0005" "\u0006" "\u0007"] -> w199
                frame 0, Default {
                }
                frame 1 {
                }
                frame 2 {
                }
                frame 3 {
                }
                frame 4 {
                }
                frame 5 {
                }
                frame 6 {
                }
                frame 7 {
                }
              }
              n64 = Concatenate Strings(w201, w199) -> (w200:string)
            }
            n65 = Bundle By Name(cluster=w175, "pibs_clstr.sens_type_1"=w174, "pibs_clstr.sens_type_2"=w173, "pibs_clstr.sens_type_3"=w172, "pibs_clstr.sens_type_4"=w171, "pibs_clstr.sens_type_5"=w170, "pibs_clstr.sens_type_6"=w169, "pibs_clstr.sens_type_7"=w168, "pibs_clstr.sens_type_8"=w167) -> (w166:T17)
            n66 = Concatenate Strings("\t" ("string"), w187) -> (w178:string)
            n67 = Bundle By Name(cluster=w165, "rs232_data_clstr.sens_type_arry"=w163) -> (w164:T14)
            n68 = VISA Write(VISA resource name=w195, write buffer=w178, error in (no error)=w193) -> (VISA resource name out=w196:refnum<visa-resource-name>, error out=w197:errorcluster)  [unwired: 1 out]
            n69 = flat-sequence {
              tunnel: w197 -> [w212]
              tunnel: [w212] -> w186
              tunnel: w196 -> [w211]
              tunnel: [w211] -> w184
              tunnel: w191 -> [w210]
              frame #0 {
                n70 = Wait (ms)(milliseconds to wait=w210) -> ()  [unwired: 1 out]
              }
            }
            n71 = property class="Instr"(reference=w184, error in=w186) -> (reference out=w183:refnum<visa-resource-name>, error out=w185:errorcluster, "Serial Settings:Number of Bytes at Serial Port"=w180:u32)
            n72 = VISA Read(VISA resource name=w183, byte count=w180, error in (no error)=w185) -> (VISA resource name out=w182:refnum<visa-resource-name>, read buffer=w177:string, return count=w179:u32, error out=w181:errorcluster)
            n73 = Bundle By Name(cluster=w166, "states"=states_cntrl."idle", "pibs_clstr.sens_typ_str"=w178, "pibs_clstr.sens_typ_str _2"=w177) -> (w190:T17)
            n74 = local write "bytes read"(w179) -> ()
            n75 = Enqueue Element(queue=w194, element=w190, error in (no error)=w181) -> ()  [unwired: 1 in, 3 out]
          }
          frame "send_cmd" {
            n76 = Unbundle By Name(w215) -> ("sens_type_arry"=w214:T6)
            n77 = local read "wr_buffr"() -> (w217:string)
            n78 = for {
              tunnel: w214 -> [w230] mode=indexing
              shift-right: [w229] -> w218
              shift-left: "" -> [w231]
              n79 = case shown="0, Default" w230 {
                tunnel: ["\u0000" "\u0001" "\u0002" "\u0003" "\u0004" "\u0005" "\u0006" "\u0007"] -> w228
                frame 0, Default {
                }
                frame 1 {
                }
                frame 2 {
                }
                frame 3 {
                }
                frame 4 {
                }
                frame 5 {
                }
                frame 6 {
                }
                frame 7 {
                }
              }
              n80 = Concatenate Strings(w231, w228) -> (w229:string)
            }
            n81 = Concatenate Strings(w217, w218) -> (w216:string)
            n82 = Bundle By Name(cluster=w220, "states"=states_cntrl."capt_wait") -> (w221:T17)
            n83 = VISA Write(VISA resource name=w227, write buffer=w216, error in (no error)=w226) -> (VISA resource name out=w225:refnum<visa-resource-name>, error out=w222:errorcluster)  [unwired: 1 out]
            n84 = Enqueue Element(queue=w223, element=w221, error in (no error)=w222) -> ()  [unwired: 1 in, 3 out]
          }
          frame "capt_wait" {
            n85 = Bundle By Name(cluster=w241, "states"=states_cntrl."read_data") -> (w242:T17)
            n86 = flat-sequence {
              tunnel: w248 -> [w252]
              tunnel: [w252] -> w244
              tunnel: w249 -> [w251]
              tunnel: [w251] -> w247
              tunnel: w243 -> [w250]
              frame #0 {
                n87 = Wait (ms)(milliseconds to wait=w250) -> ()  [unwired: 1 out]
              }
            }
            n88 = Enqueue Element(queue=w245, element=w242, error in (no error)=w244) -> ()  [unwired: 1 in, 3 out]
          }
          frame "read_data" {
            n89 = property class="Instr"(reference=w262, error in=w261) -> (reference out=w264:refnum<visa-resource-name>, error out=w263:errorcluster, "Serial Settings:Number of Bytes at Serial Port"=w256:u32)
            n90 = VISA Read(VISA resource name=w264, byte count=w256, error in (no error)=w263) -> (VISA resource name out=w260:refnum<visa-resource-name>, read buffer=w257:string, return count=w258:u32, error out=w259:errorcluster)
            n91 = Bundle By Name(cluster=w254, "states"=states_cntrl."chk_bytes_rd", "bytes read"=w258, "Response"=w257, "bytes_at_port"=w256) -> (w255:T17)
            n92 = Enqueue Element(queue=w265, element=w255, error in (no error)=w259) -> ()  [unwired: 1 in, 3 out]
          }
          frame "chk_bytes_rd" {
            (unwired) u32 56 ("y")
            # "Only display data\nif we have received\n56 bytes of data."
            n93 = Unbundle By Name(w269) -> ("bytes read"=w275:u32)
            n94 = local read "chk_bytes_rd"() -> (w267:u32)
            n95 = Equal?(x=w275, y=w267) -> (x = y?=w274:bool)
            n96 = Select(t=states_cntrl."disp_data" ("states"), s=w274, f=states_cntrl."small_dwell") -> (s? t:f=w271:T9)
            n97 = Bundle By Name(cluster=w269, "states"=w271) -> (w270:T17)
            n98 = Enqueue Element(queue=w278, element=w270, error in (no error)=w276) -> ()  [unwired: 1 in, 3 out]
          }
          frame "disp_data" {
            n99 = local read "minor_qsm_qry"() -> (w282:bool)
            n100 = Select(t=w281, s=w282, f=w280) -> (s? t:f=w279:T17)
            n101 = while {
              shift-right: [w314] -> w284
              shift-left: w279 -> [w313]
              tunnel: w285 -> [w311]
              i -> [w299]
              stop <- w296 stop-if-true
              w305 = -1 ("y")
              w302 = 0 ("offset (0)")
              (unwired) "á" ("format string")
              n102 = Unbundle By Name(w313) -> ("Response"=w304:string, "log_tabl_row_cnt"=w309:u64, "above_row_7"=w310:bool, "sens_type_arry"=w300:T6)
              n103 = Index Array(array=w300, index=w299) -> (element=w298:T2)
              n104 = case shown="1" w298 {
                tunnel: ["á" ("format string") "‰" ("format string")] -> w297
                tunnel: [3 ("offset (0)") 0 ("offset (0)")] -> w295
                frame 0, Default {
                }
                frame 1 {
                }
              }
              n105 = Match Pattern(string=w304, regular expression=w297, offset (0)=w302) -> (after substring=w315:string, offset past match=w317:i32)  [unwired: 2 out]
              n106 = Match Pattern(string=w304, regular expression="‰" ("format string"), offset (0)=w302) -> (offset past match=w306:i32)  [unwired: 3 out]
              n107 = Select(t=u64 0, s=w310, f=w309) -> (s? t:f=w307:u64)
              n108 = Equal?(x=w317, y=w305) -> (x = y?=w296:bool)
              n109 = Equal?(x=w306, y=w305) -> (x = y?=w301:bool)
              n110 = And(x=w296, y=w301) -> ()  [unwired: 1 out]
              n111 = String Subset(string=w315, offset (0)=w302, length (rest)=6 ("length (rest)")) -> (substring=w316:string)
              n112 = case shown="False" w296 {
                tunnel: w316 -> [w331 _]
                tunnel: w299 -> [w332 _]
                tunnel: w313 -> [w329 w505]
                tunnel: [w328 w505] -> w312
                tunnel: w311 -> [w327 _]
                tunnel: w307 -> [w326 _]
                tunnel: w310 -> [w325 _]
                tunnel: w298 -> [w324 _]
                tunnel: w295 -> [w323 _]
                frame False {
                  n113 = case shown="0, Default" w332 {
                    selector: w332 -> [w346 w371 w389 w407 w425 w444 w464 w489]
                    tunnel: w331 -> [w339 w363 w384 w403 w422 w441 w460 w477]
                    tunnel: w323 -> [w359 w378 w397 w416 w435 w454 w473 w496]
                    tunnel: 2 ("length (rest)") -> [w358 w377 w396 w415 w434 w453 w472 w495]
                    tunnel: w329 -> [w340 w376 w395 w414 w433 w452 w471 w494]
                    tunnel: [w333 w360 w379 w398 w417 w436 w456 w474] -> w328
                    tunnel: w327 -> [_ _ _ _ _ _ _ _]
                    tunnel: w326 -> [w343 w372 w388 w406 w426 w445 w465 w485]
                    tunnel: w325 -> [w342 w373 w390 w409 w427 w447 w466 w484]
                    tunnel: w324 -> [w341 w366 w385 w404 w423 w442 w461 w482]
                    frame 0, Default {
                      w352 = 0 ("tableIndx")
                      n114 = Increment(x=w346) -> (x+1=w345:i32)
                      n115 = call "conv_temp.vi"("sens_type"=w341, "length (rest)"=w358, "offset (0)"=w359, "Response"=w339) -> ("rh"=w337:T3, "f_temp"=w338:T4)  [unwired: 6 in]
                      n116 = Get Date/Time String(want seconds? (F)=TRUE) -> (date string=w351:string, time string=w350:string)  [unwired: 2 in]
                      n117 = call "fill_sens_dat.vi"("f_temp"=w338, "rh_0"=w337, "raw_dat"=w339, "index"=w346, "element in"=w340) -> ("element out"=w335:T17)  [unwired: 6 in]
                      n118 = Concatenate Strings(w351, "," ("string"), w350) -> (w336:string)
                      n119 = Unbundle By Name(w335) -> ("logTable in"=w354:string[][][])
                      n120 = call "log_table_first_row_in_push_down_rest.vi"("String"=w351, "tableIndx"=w352, "colIndx"=w346, "insertRow"=w343, "pass8thRow"=w342, "logTable in"=w354) -> ("logTable out"=w353:string[][][])  [unwired: 5 in]
                      n121 = call "log_table_first_row_in_push_down_rest.vi"("String"=w350, "tableIndx"=w352, "colIndx"=w345, "insertRow"=w343, "pass8thRow"=w342, "logTable in"=w353) -> ("logTable out"=w355:string[][][])  [unwired: 5 in]
                      n122 = Number To Fractional String(number=w338, width (-)=i16 5, precision (6)=i16 2) -> (F-format string=w347:string)  [unwired: 1 in]
                      n123 = Increment(x=w345) -> (x+1=w344:i32)
                      n124 = call "log_table_first_row_in_push_down_rest.vi"("String"=w347, "tableIndx"=w352, "colIndx"=w344, "insertRow"=w343, "pass8thRow"=w342, "logTable in"=w355) -> ("logTable out"=w334:string[][][])  [unwired: 5 in]
                      n125 = Bundle By Name(cluster=w335, "pibs_clstr.sen_1"=w339, "pibs_clstr.sen_1_num"=w338, "pibs_clstr.rh_1"=w337, "dts"=w336, "temp_clstr.dts"=w336, "logTable in"=w334) -> (w333:T17)
                    }
                    frame 1 {
                      n126 = call "conv_temp.vi"("sens_type"=w366, "length (rest)"=w377, "offset (0)"=w378, "Response"=w363) -> ("rh"=w361:T3, "f_temp"=w362:T4)  [unwired: 6 in]
                      n127 = call "fill_sens_dat.vi"("f_temp"=w362, "rh_0"=w361, "raw_dat"=w363, "index"=w371, "element in"=w376) -> ("element out"=w364:T17)  [unwired: 6 in]
                      n128 = Unbundle By Name(w364) -> ("logTable in"=w375:string[][][])
                      n129 = Number To Fractional String(number=w362, width (-)=i16 5, precision (6)=i16 2) -> (F-format string=w368:string)  [unwired: 1 in]
                      n130 = call "log_table_first_row_in_push_down_rest.vi"("String"=w368, "tableIndx"=0, "colIndx"=3, "insertRow"=w372, "pass8thRow"=w373, "logTable in"=w375) -> ("logTable out"=w365:string[][][])  [unwired: 5 in]
                      n131 = Bundle By Name(cluster=w364, "pibs_clstr.sen_2"=w363, "pibs_clstr.sen_2_num"=w362, "pibs_clstr.rh_2"=w361, "logTable in"=w365) -> (w360:T17)
                    }
                    frame 2 {
                      n132 = call "conv_temp.vi"("sens_type"=w385, "length (rest)"=w396, "offset (0)"=w397, "Response"=w384) -> ("rh"=w382:T3, "f_temp"=w383:T4)  [unwired: 6 in]
                      n133 = call "fill_sens_dat.vi"("f_temp"=w383, "rh_0"=w382, "raw_dat"=w384, "index"=w389, "element in"=w395) -> ("element out"=w380:T17)  [unwired: 6 in]
                      n134 = Unbundle By Name(w380) -> ("logTable in"=w394:string[][][])
                      n135 = Number To Fractional String(number=w383, width (-)=i16 5, precision (6)=i16 2) -> (F-format string=w391:string)  [unwired: 1 in]
                      n136 = call "log_table_first_row_in_push_down_rest.vi"("String"=w391, "tableIndx"=0, "colIndx"=4, "insertRow"=w388, "pass8thRow"=w390, "logTable in"=w394) -> ("logTable out"=w381:string[][][])  [unwired: 5 in]
                      n137 = Bundle By Name(cluster=w380, "pibs_clstr.sen_3"=w384, "pibs_clstr.sen_3_num"=w383, "pibs_clstr.rh_3"=w382, "logTable in"=w381) -> (w379:T17)
                    }
                    frame 3 {
                      n138 = call "conv_temp.vi"("sens_type"=w404, "length (rest)"=w415, "offset (0)"=w416, "Response"=w403) -> ("rh"=w401:T3, "f_temp"=w402:T4)  [unwired: 6 in]
                      n139 = call "fill_sens_dat.vi"("f_temp"=w402, "rh_0"=w401, "raw_dat"=w403, "index"=w407, "element in"=w414) -> ("element out"=w399:T17)  [unwired: 6 in]
                      n140 = Unbundle By Name(w399) -> ("logTable in"=w413:string[][][])
                      n141 = Number To Fractional String(number=w402, width (-)=i16 5, precision (6)=i16 2) -> (F-format string=w410:string)  [unwired: 1 in]
                      n142 = call "log_table_first_row_in_push_down_rest.vi"("String"=w410, "tableIndx"=0, "colIndx"=5, "insertRow"=w406, "pass8thRow"=w409, "logTable in"=w413) -> ("logTable out"=w400:string[][][])  [unwired: 5 in]
                      n143 = Bundle By Name(cluster=w399, "pibs_clstr.sen_4"=w403, "pibs_clstr.sen_4_num"=w402, "pibs_clstr.rh_4"=w401, "logTable in"=w400) -> (w398:T17)
                    }
                    frame 4 {
                      n144 = call "conv_temp.vi"("sens_type"=w423, "length (rest)"=w434, "offset (0)"=w435, "Response"=w422) -> ("rh"=w420:T3, "f_temp"=w421:T4)  [unwired: 6 in]
                      n145 = call "fill_sens_dat.vi"("f_temp"=w421, "rh_0"=w420, "raw_dat"=w422, "index"=w425, "element in"=w433) -> ("element out"=w418:T17)  [unwired: 6 in]
                      n146 = Unbundle By Name(w418) -> ("logTable in"=w432:string[][][])
                      n147 = Number To Fractional String(number=w421, width (-)=i16 5, precision (6)=i16 2) -> (F-format string=w429:string)  [unwired: 1 in]
                      n148 = call "log_table_first_row_in_push_down_rest.vi"("String"=w429, "tableIndx"=0, "colIndx"=6, "insertRow"=w426, "pass8thRow"=w427, "logTable in"=w432) -> ("logTable out"=w419:string[][][])  [unwired: 5 in]
                      n149 = Bundle By Name(cluster=w418, "pibs_clstr.sen_5"=w422, "pibs_clstr.sen_5_num"=w421, "pibs_clstr.rh_5"=w420, "logTable in"=w419) -> (w417:T17)
                    }
                    frame 5 {
                      n150 = call "conv_temp.vi"("sens_type"=w442, "length (rest)"=w453, "offset (0)"=w454, "Response"=w441) -> ("rh"=w439:T3, "f_temp"=w440:T4)  [unwired: 6 in]
                      n151 = call "fill_sens_dat.vi"("f_temp"=w440, "rh_0"=w439, "raw_dat"=w441, "index"=w444, "element in"=w452) -> ("element out"=w437:T17)  [unwired: 6 in]
                      n152 = Unbundle By Name(w437) -> ("logTable in"=w451:string[][][])
                      n153 = Number To Fractional String(number=w440, width (-)=i16 5, precision (6)=i16 2) -> (F-format string=w448:string)  [unwired: 1 in]
                      n154 = call "log_table_first_row_in_push_down_rest.vi"("String"=w448, "tableIndx"=0, "colIndx"=7, "insertRow"=w445, "pass8thRow"=w447, "logTable in"=w451) -> ("logTable out"=w438:string[][][])  [unwired: 5 in]
                      n155 = Bundle By Name(cluster=w437, "pibs_clstr.sen_6"=w441, "pibs_clstr.sen_6_num"=w440, "pibs_clstr.rh_6"=w439, "logTable in"=w438) -> (w436:T17)
                    }
                    frame 6 {
                      n156 = call "conv_temp.vi"("sens_type"=w461, "length (rest)"=w472, "offset (0)"=w473, "Response"=w460) -> ("rh"=w458:T3, "f_temp"=w459:T4)  [unwired: 6 in]
                      n157 = call "fill_sens_dat.vi"("f_temp"=w459, "rh_0"=w458, "raw_dat"=w460, "index"=w464, "element in"=w471) -> ("element out"=w455:T17)  [unwired: 6 in]
                      n158 = Unbundle By Name(w455) -> ("logTable in"=w470:string[][][])
                      n159 = Number To Fractional String(number=w459, width (-)=i16 5, precision (6)=i16 2) -> (F-format string=w467:string)  [unwired: 1 in]
                      n160 = call "log_table_first_row_in_push_down_rest.vi"("String"=w467, "tableIndx"=0, "colIndx"=8, "insertRow"=w465, "pass8thRow"=w466, "logTable in"=w470) -> ("logTable out"=w457:string[][][])  [unwired: 5 in]
                      n161 = Bundle By Name(cluster=w455, "pibs_clstr.sen_7"=w460, "pibs_clstr.sen_7_num"=w459, "pibs_clstr.rh_7"=w458, "logTable in"=w457) -> (w456:T17)
                    }
                    frame 7 {
                      n162 = call "conv_temp.vi"("sens_type"=w482, "length (rest)"=w495, "offset (0)"=w496, "Response"=w477) -> ("rh"=w475:T3, "f_temp"=w476:T4)  [unwired: 6 in]
                      n163 = call "fill_sens_dat.vi"("f_temp"=w476, "rh_0"=w475, "raw_dat"=w477, "index"=w489, "element in"=w494) -> ("element out"=w478:T17)  [unwired: 6 in]
                      n164 = case shown="False" w484 {
                        selector: w484 -> [w497 w503]
                        tunnel: [w501 w503] -> w479
                        tunnel: [w500 w504] -> w480
                        tunnel: w485 -> [w499 w504]
                        frame False {
                          (unwired) i16 2 ("precision (6)")
                          n165 = Increment(x=w499) -> (x+1=w498:u64)
                          n166 = Greater?(x=w498, y=u64 6) -> (0:w501:bool)
                          n167 = Select(t=w499, s=w497, f=w498) -> (s? t:f=w500:u64)
                        }
                        frame True {
                        }
                      }
                      n168 = Unbundle By Name(w478) -> ("logTable in"=w493:string[][][])
                      n169 = Number To Fractional String(number=w476, width (-)=i16 5, precision (6)=i16 2) -> (F-format string=w491:string)  [unwired: 1 in]
                      n170 = call "log_table_first_row_in_push_down_rest.vi"("String"=w491, "tableIndx"=0, "colIndx"=9, "insertRow"=w485, "pass8thRow"=w484, "logTable in"=w493) -> ("logTable out"=w481:string[][][])  [unwired: 5 in]
                      n171 = Bundle By Name(cluster=w478, "pibs_clstr.sen_8"=w477, "pibs_clstr.sen_8_num"=w476, "pibs_clstr.rh_8"=w475, "logTable in"=w481, "log_tabl_row_cnt"=w480, "above_row_7"=w479) -> (w474:T17)
                      n172 = Index Array(array=w481, index (dim 0)=0 ("index (page)")) -> (element=w487:string[][])  [unwired: 2 in]
                      n173 = property on="mult_list" class="MCListbox (strict)"("ItemNames"=w487) -> ()  [unwired: 2 in, 2 out]
                    }
                  }
                }
                frame True {
                }
              }
              n174 = Bundle By Name(cluster=w312, "Response"=w315) -> (w314:T17)
            }
            n175 = Unbundle By Name(w279) -> ("bytes read"=w289:u32, "Response"=w290:string, "bytes_at_port"=w291:u32)
            n176 = local write "bytes read"(w289) -> ()
            n177 = local write "Response"(w290) -> ()
            n178 = local write "bytes_at_port"(w291) -> ()
            n179 = Bundle By Name(cluster=w284, "states"=states_cntrl."sav_qry") -> (w288:T17)
            n180 = Enqueue Element(queue=w294, element=w288, error in (no error)=w292) -> (error out=w286:errorcluster)  [unwired: 1 in, 2 out]
          }
          frame "sav_qry" {
            n181 = local read "Save"() -> (w516:bool)
            n182 = Select(t=states_cntrl."sav_dat" ("states"), s=w516, f=states_cntrl."dwell") -> (s? t:f=w512:T9)
            n183 = Bundle By Name(cluster=w513, "states"=w512) -> (w510:T17)
            n184 = Enqueue Element(queue=w511, element=w510, error in (no error)=w509) -> (error out=w508:errorcluster)  [unwired: 1 in, 2 out]
          }
          frame "sav_dat" {
            n185 = local read "Save"() -> (w517:bool)
            n186 = case shown="True" w517 {
              tunnel: w519 -> [_ w545]
              frame False {
              }
              frame True {
                w529 = "," ("string")
                w532 = "%5.2f" ("format string")
                w531 = "," ("delimiter (Tab)")
                n187 = Unbundle By Name(w545) -> ("temp_clstr"=w544:T18)
                n188 = Unbundle By Name(w544) -> ("dts"=w543:string, "temp_f_arry"=w537:T4[], "sens_dat_raw_arry"=w536:string[], "rh_arry"=w533:T19)
                n189 = for {
                  tunnel: w537 -> [w552] mode=indexing
                  shift-right: [w551] -> _
                  shift-left: "" -> [w550]
                  tunnel: w536 -> [w546] mode=indexing
                  w548 = "," ("string")
                  n190 = Number To Fractional String(number=w552, width (-)=i16 5) -> (F-format string=w549:string)  [unwired: 2 in]
                  n191 = Concatenate Strings(w550, w548, w549, w548, w546) -> (w551:string)
                }
                n192 = Array To Spreadsheet String(delimiter (Tab)=w531, array=w537, 3:w532) -> (spreadsheet string=w535:string)
                n193 = Array To Spreadsheet String(delimiter (Tab)=w531, array=w533, 3:w532) -> (spreadsheet string=w530:string)
                n194 = local read "Path"() -> (w540:path)
                n195 = Concatenate Strings(w543, w529, w535, w529, w530, "\n") -> (w541:string)
                "concatenated string" <- w541
                n196 = Get File Size(file=w540) -> (refnum out=w539:refnum<file>, 0:w527:errorcluster)  [unwired: 1 in, 1 out]
                n197 = Set File Position(refnum=w539, from (0:start)=enum16{"start", "end", "current"}."end", error in=w527) -> (refnum out=w538:refnum<file>, error out=w526:errorcluster)  [unwired: 1 in]
                n198 = Write to Text File(file (use dialog)=w538, text=w541, error in=w526) -> ()  [unwired: 1 in, 3 out]
              }
            }
            n199 = Bundle By Name(cluster=w519, "states"=states_cntrl."dwell" ("f")) -> (w524:T17)
            n200 = Enqueue Element(queue=w525, element=w524, error in (no error)=w523) -> (error out=w522:errorcluster)  [unwired: 1 in, 2 out]
          }
          frame "dwell" {
            n201 = local read "dwell_s"() -> (w553:u32)
            n202 = Multiply(x=w553, y=u32 1000) -> (x*y=w558:u32)
            n203 = Bundle By Name(cluster=w555, "states"=states_cntrl."stop_capt_qry") -> (w556:T17)
            n204 = flat-sequence {
              tunnel: w563 -> [w566]
              tunnel: [w566] -> w559
              tunnel: w564 -> [w565]
              tunnel: [w565] -> w562
              tunnel: w558 -> [w567]
              frame #0 {
                n205 = Wait (ms)(milliseconds to wait=w567) -> ()  [unwired: 1 out]
              }
            }
            n206 = Enqueue Element(queue=w560, element=w556, error in (no error)=w559) -> ()  [unwired: 1 in, 3 out]
          }
          frame "small_dwell" {
            n207 = local read "small_dwell"() -> (w568:u32)
            n208 = Multiply(x=w568, y=u32 1000) -> (x*y=w573:u32)
            n209 = Bundle By Name(cluster=w570, "states"=states_cntrl."stop_capt_qry") -> (w571:T17)
            n210 = flat-sequence {
              tunnel: w578 -> [w581]
              tunnel: [w581] -> w574
              tunnel: w579 -> [w580]
              tunnel: [w580] -> w577
              tunnel: w573 -> [w582]
              frame #0 {
                n211 = Wait (ms)(milliseconds to wait=w582) -> ()  [unwired: 1 out]
              }
            }
            n212 = Enqueue Element(queue=w575, element=w571, error in (no error)=w574) -> ()  [unwired: 1 in, 3 out]
          }
          frame "stop_capt_qry" {
            n213 = local read "minor_qsm_qry"() -> (w586:bool)
            n214 = local read "auto_capt_data"() -> (w590:bool)
            n215 = Select(t=states_cntrl."go_to_minor_qsm" ("states"), s=w586, f=states_cntrl."send_cmd" ("states")) -> (s? t:f=w583:T9)
            n216 = Select(t=w583, s=w590, f=states_cntrl."idle") -> (s? t:f=w592:T9)
            n217 = Bundle By Name(cluster=w588, "states"=w592) -> (w589:T17)
            n218 = Enqueue Element(queue=w595, element=w589, error in (no error)=w593) -> ()  [unwired: 1 in, 3 out]
          }
        }
      }
      frame Error {
        # "Return true in any case that should stop the loop."
      }
    }
    n219 = Unbundle By Name(w34) -> ("pibs_clstr"=w33:T12)
    n220 = local write "pibs_clstr"(w33) -> ()
  }
  n221 = call "rs232_qsm.vi"() -> ()  [unwired: 12 in]
  n222 = while {
    shift-right: [w608] -> w28
    shift-left: w29 -> [w610]
    tunnel: w16 -> [w611]
    tunnel: w12 -> [w604]
    shift-right: [w603] -> _
    shift-left: w5 -> [w605]
    tunnel: w6 -> [w602]
    shift-left: w5 -> [w601]
    stop <- w606 stop-if-true
    # "This loop is the producer loop."
    n223 = event shown="[11] \"capt_data\": Value Change" {
      selector: w604 -> [_ _ _ _ _ _ _ _ _ _ _ _ _ _]
      dyn-events: _ -> [_ _ _ _ _ _ _ _ _ _ _ _ _ _]
      timeout: _ -> [_ _ _ _ _ _ _ _ _ _ _ _ _ _]
      tunnel: w611 -> [w615 _ w639 _ _ _ _ _ _ _ _ w733 w751 _]
      tunnel: w610 -> [w612 w630 w638 w648 w658 w668 w678 w688 w698 w708 w718 w732 w750 w766]
      tunnel: [w613 w630 w637 w648 w658 w668 w678 w688 w698 w708 w718 w731 w749 w765] -> w608
      tunnel: ["stop" FALSE ("stop") FALSE ("stop") FALSE ("stop") FALSE ("stop") FALSE ("stop") FALSE ("stop") FALSE ("stop") FALSE ("stop") FALSE ("stop") FALSE ("stop") FALSE ("stop") FALSE ("stop") FALSE ("stop")] -> w609
      tunnel: w605 -> [w614 w628 w640 w654 w664 w674 w684 w694 w704 w714 w724 w729 w747 w763]
      tunnel: [w614 w627 w636 w650 w660 w670 w680 w690 w700 w710 w720 w728 w746 w763] -> w603
      tunnel: w602 -> [_ _ _ w656 w666 w676 w686 w696 w706 w716 w726 _ _ _]
      tunnel: w601 -> [_ _ w634 _ _ _ _ _ _ _ _ _ _ _]
      event "stop": Value Change {
        n224 = event-data() -> ()  [unwired: 1 in, 1 out]
        n225 = Bundle By Name(cluster=w614, "states"=states_cntrl."exit") -> (w616:T17)
        n226 = Enqueue Element(queue=w615, element=w616, error in (no error)=w612) -> (error out=w613:errorcluster)  [unwired: 1 in, 2 out]
      }
      event User Event {
        # "updates from initialize state below"
        n227 = event-data() -> ("states"=w626:T9, "temp_clstr"=w625:T18, "logTable in"=w624:string[][][], "log_tabl_row_cnt"=w623:u64, "above_row_7"=w622:bool, "temp_clstr.temp_f_arry"=w621:T4[], "temp_clstr.rh_arry"=w620:T19, "sens_type_arry"=w619:T6)  [unwired: 1 in]
        n228 = Bundle By Name(cluster=w628, "states"=w626, "temp_clstr"=w625, "logTable in"=w624, "log_tabl_row_cnt"=w623, "above_row_7"=w622, "temp_clstr.temp_f_arry"=w621, "temp_clstr.rh_arry"=w620, "sens_type_arry"=w619) -> (w627:T17)
      }
      event User Event {
        n229 = event-data() -> ()  [unwired: 1 in, 1 out]
        n230 = Unbundle By Name(w640) -> ("sens_type_arry"=w631:T6)
        n231 = Unbundle By Name(w634) -> ("sens_type_arry"=w633:T6)
        n232 = Not Equal?(x=w631, y=w633) -> (x != y?=w632:bool)
        n233 = Bundle By Name(cluster=w640, "sens_type_arry"=w631, "states"=states_cntrl."snd_sens_type") -> (w636:T17)
        n234 = case shown="True" w632 {
          tunnel: w639 -> [_ w646]
          tunnel: w638 -> [w642 w645]
          tunnel: [w642 w644] -> w637
          tunnel: w636 -> [_ w643]
          frame False {
          }
          frame True {
            n235 = Enqueue Element(queue=w646, element=w643, error in (no error)=w645) -> (error out=w644:errorcluster)  [unwired: 1 in, 2 out]
          }
        }
      }
      event Value Change {
        n236 = event-data() -> ("NewVal"=w651:T2)  [unwired: 1 in]
        n237 = Unbundle By Name(w656) -> ("regEvntSenTyp"=w655:refnum<user-event>)
        n238 = Unbundle By Name(w654) -> ("sens_type_arry"=w653:T6)
        n239 = Generate User Event(user event=w655, event data cluster=w651) -> ()  [unwired: 2 in, 2 out]
        n240 = Replace Array Subset(array=w653, new element=w651, index=0) -> (w649:T6)
        n241 = Bundle By Name(cluster=w654, "sens_type_arry"=w649) -> (w650:T17)
      }
      event Value Change {
        n242 = event-data() -> ("NewVal"=w661:T2)  [unwired: 1 in]
        n243 = Unbundle By Name(w666) -> ("regEvntSenTyp"=w665:refnum<user-event>)
        n244 = Unbundle By Name(w664) -> ("sens_type_arry"=w663:T6)
        n245 = Generate User Event(user event=w665, event data cluster=w661) -> ()  [unwired: 2 in, 2 out]
        n246 = Replace Array Subset(array=w663, new element=w661, index=1) -> (w659:T6)
        n247 = Bundle By Name(cluster=w664, "sens_type_arry"=w659) -> (w660:T17)
      }
      event Value Change {
        n248 = event-data() -> ("NewVal"=w671:T2)  [unwired: 1 in]
        n249 = Unbundle By Name(w676) -> ("regEvntSenTyp"=w675:refnum<user-event>)
        n250 = Unbundle By Name(w674) -> ("sens_type_arry"=w673:T6)
        n251 = Generate User Event(user event=w675, event data cluster=w671) -> ()  [unwired: 2 in, 2 out]
        n252 = Replace Array Subset(array=w673, new element=w671, index=2) -> (w669:T6)
        n253 = Bundle By Name(cluster=w674, "sens_type_arry"=w669) -> (w670:T17)
      }
      event Value Change {
        n254 = event-data() -> ("NewVal"=w681:T2)  [unwired: 1 in]
        n255 = Unbundle By Name(w686) -> ("regEvntSenTyp"=w685:refnum<user-event>)
        n256 = Unbundle By Name(w684) -> ("sens_type_arry"=w683:T6)
        n257 = Generate User Event(user event=w685, event data cluster=w681) -> ()  [unwired: 2 in, 2 out]
        n258 = Replace Array Subset(array=w683, new element=w681, index=3) -> (w679:T6)
        n259 = Bundle By Name(cluster=w684, "sens_type_arry"=w679) -> (w680:T17)
      }
      event Value Change {
        n260 = event-data() -> ("NewVal"=w691:T2)  [unwired: 1 in]
        n261 = Unbundle By Name(w696) -> ("regEvntSenTyp"=w695:refnum<user-event>)
        n262 = Unbundle By Name(w694) -> ("sens_type_arry"=w693:T6)
        n263 = Generate User Event(user event=w695, event data cluster=w691) -> ()  [unwired: 2 in, 2 out]
        n264 = Replace Array Subset(array=w693, new element=w691, index=4) -> (w689:T6)
        n265 = Bundle By Name(cluster=w694, "sens_type_arry"=w689) -> (w690:T17)
      }
      event Value Change {
        n266 = event-data() -> ("NewVal"=w701:T2)  [unwired: 1 in]
        n267 = Unbundle By Name(w706) -> ("regEvntSenTyp"=w705:refnum<user-event>)
        n268 = Unbundle By Name(w704) -> ("sens_type_arry"=w703:T6)
        n269 = Generate User Event(user event=w705, event data cluster=w701) -> ()  [unwired: 2 in, 2 out]
        n270 = Replace Array Subset(array=w703, new element=w701, index=5) -> (w699:T6)
        n271 = Bundle By Name(cluster=w704, "sens_type_arry"=w699) -> (w700:T17)
      }
      event Value Change {
        n272 = event-data() -> ("NewVal"=w711:T2)  [unwired: 1 in]
        n273 = Unbundle By Name(w716) -> ("regEvntSenTyp"=w715:refnum<user-event>)
        n274 = Unbundle By Name(w714) -> ("sens_type_arry"=w713:T6)
        n275 = Generate User Event(user event=w715, event data cluster=w711) -> ()  [unwired: 2 in, 2 out]
        n276 = Replace Array Subset(array=w713, new element=w711, index=6) -> (w709:T6)
        n277 = Bundle By Name(cluster=w714, "sens_type_arry"=w709) -> (w710:T17)
      }
      event Value Change {
        n278 = event-data() -> ("NewVal"=w721:T2)  [unwired: 1 in]
        n279 = Unbundle By Name(w726) -> ("regEvntSenTyp"=w725:refnum<user-event>)
        n280 = Unbundle By Name(w724) -> ("sens_type_arry"=w723:T6)
        n281 = Generate User Event(user event=w725, event data cluster=w721) -> ()  [unwired: 2 in, 2 out]
        n282 = Replace Array Subset(array=w723, new element=w721, index=7) -> (w719:T6)
        n283 = Bundle By Name(cluster=w724, "sens_type_arry"=w719) -> (w720:T17)
      }
      event "capt_data": Value Change {
        # "Go to state capt_data below\nand capture data."
        n284 = event-data() -> ("NewVal"=w727:bool)  [unwired: 1 in]
        n285 = case shown="True" w727 {
          tunnel: w733 -> [_ w744]
          tunnel: w732 -> [w734 w743]
          tunnel: [w734 w742] -> w731
          tunnel: w729 -> [w735 w741]
          tunnel: [w735 w740] -> w728
          frame False {
          }
          frame True {
            n286 = local read "minor_qsm_qry"() -> (w739:bool)
            n287 = Select(t=states_cntrl."go_to_minor_qsm" ("states"), s=w739, f=states_cntrl."capt_data") -> (s? t:f=w736:T9)
            n288 = Bundle By Name(cluster=w741, "states"=w736) -> (w740:T17)
            n289 = Enqueue Element(queue=w744, element=w740, error in (no error)=w743) -> (error out=w742:errorcluster)  [unwired: 1 in, 2 out]
          }
        }
      }
      event "auto_capt_data": Value Change {
        n290 = event-data() -> ("NewVal"=w745:bool)  [unwired: 1 in]
        n291 = case shown="True" w745 {
          tunnel: w751 -> [_ w762]
          tunnel: w750 -> [w752 w761]
          tunnel: [w752 w760] -> w749
          tunnel: w747 -> [w753 w759]
          tunnel: [w753 w758] -> w746
          frame False {
          }
          frame True {
            n292 = local read "minor_qsm_qry"() -> (w757:bool)
            n293 = Select(t=states_cntrl."go_to_minor_qsm" ("states"), s=w757, f=states_cntrl."send_cmd" ("states")) -> (s? t:f=w754:T9)
            n294 = Bundle By Name(cluster=w759, "states"=w754) -> (w758:T17)
            n295 = Enqueue Element(queue=w762, element=w758, error in (no error)=w761) -> (error out=w760:errorcluster)  [unwired: 1 in, 2 out]
          }
        }
      }
      event "create_file": Value Change {
        n296 = event-data() -> ()  [unwired: 1 in, 5 out]
        n297 = Open/Create/Replace File(file path (use dialog)="Path", error in=w766, operation (0:open)=T20."create", access (0:read/write)=enum16{"read/write", "read-only", "write-only"}."read/write") -> (error out=w765:errorcluster)  [unwired: 2 in, 2 out]
      }
    }
    n298 = Unbundle By Name(w608) -> ("status"=w607:bool)
    n299 = Or(x=w607, y=w609) -> (x .or. y?=w606:bool)
  }
  n300 = Release Queue(queue=w16, error in (no error)=w28) -> ()  [unwired: 1 in, 3 out]
  n301 = VISA Close(VISA resource name=w19, error in (no error)=w18) -> (error out=w20:errorcluster)
  n302 = call <vilib>:"Simple Error Handler.vi"("error in (no error)"=w20) -> ()  [unwired: 1 in, 8 out]
